vi "NewTS-ExecutionEngine.vi"() -> ()   [LabVIEW 2020]
uses:
  SubVIs/ExEng_TypeDefs.llb/ExcEng_TestCommand.ctl
  SubVIs/ExEng_TypeDefs.llb/ExecEng_LimitsType.ctl
  LabVIEW 2020 Toolkits/toolkits_lv2020_32bit/Synchronization.llb/SynchRefs_SetGet.ctl
  LabVIEW 2020 Toolkits/VI Server Toolkit/VI Server Libraries/VI Server_SetControl.llb/VI Server_1D_STR_Set.vi
  LabVIEW 2020 Toolkits/VI Server Toolkit/VI Server Libraries/VI Server_GetControl.llb/VI Server_1D_Array_STR_Get.vi
  LabVIEW 2020 Toolkits/VI Server Toolkit/VI Server Libraries/VI Server_SetControl.llb/VI Server_1D_U16_Set.vi
  LabVIEW 2020 Toolkits/VI Server Toolkit/VI Server Libraries/VI Server_GetControl.llb/VI Server_DBL_Get.vi
  LabVIEW 2020 Toolkits/VI Server Toolkit/VI Server Libraries/VI Server_Set Controls.llb/Set STR Control.vi
  LabVIEW 2020 Toolkits/VI Server Toolkit/VI Server Libraries/VI Server_GetControl.llb/VI Server_Bool_Get.vi
  LabVIEW 2020 Toolkits/VI Server Toolkit/VI Server Libraries/VI Server_SetControl.llb/VI Server_BOOL_Set.vi
  LabVIEW 2020 Toolkits/VI Server Toolkit/VI Server Libraries/VI Server_SetControl.llb/VI Server_DBL_Set.vi
  LabVIEW 2020 Toolkits/VI Server Toolkit/VI Server Libraries/VI Server_GetControl.llb/VI Server_STR_Get.vi
  LabVIEW 2020 Toolkits/VI Server Toolkit/VI Server Toolkit LV2013.lvlib
panel:
  in  "Test.PauseOnFailure":bool caption="Pause On Failure"
  in  "Test.Pause":bool
  in  "Test.Start":bool
  in  "EmergencyStop":bool
  in  "Test.ABORT":bool
  out "System.Message":string caption="System Message:"
  in  "Help":bool
  in  "EXIT":bool
  in  "Tab.Main":T1(tab)=enum."TEST EDITOR"
  out "Test.NumberOfJumps":i32 caption="Number Of Jumps"
  out "Test.Repeat.NumberOfFailures":i32 caption="Number Of Failures"
  out "Test.Repeat.RunOf":string caption="Test:Run"
  in  "SerialNumbers.Array":string[](array[string])=["sssss"] caption="Serial Numbers"
  out "Test.ElapsedTime":string="mm:ss" caption="Elapsed: Time"
  out "Test.Progress":u16(slide) caption="Progress" scale=0.0..100.0
  out "Messages & Status":string="Test Not Started"
  in  "Test.P/N":u16(ring)=4 caption="Part #" items=["BK Precision1696 Demo", "ExecEng Verification", "Execution Engive 2", "NewTS Video Demo", "NewTS Video Demo_1", "NI-USB6001", "NI-USB6343 Demo", "NI-USB6343 Demo MultiSlot", "NI-USB6525 Demo", "Operator Interface Demo", "PCIe-1760", "PIXCI-SV7", "SeaCOM-7203", "Slow drive", "SRS5330A Test", "USB 6343_test2", "USB6001 Test", "VECTOR 1610 Demo"]
  in  "Test.Tree":string[](tree) caption="Test"
  in  "TestCaseConfiguration_VisibleRow_Decr":bool
  in  "TestCaseConfiguration_VisibleRow_Incr":bool
  in  "CurrentInstruction":i32[](listbox)=[-1] caption="Current Instruction"
  in  "Test.EndTime":string caption="Test End Time"
  in  "Test.StartTime":string caption="Test Start Time"
  in  "Fixture.SlotSelector":u16(ring) caption="Fixture Slot Selector" items=["Slot 1"]
  out "TestCase.SAVE.Success":bool
  in  "TestCase.Update.Instruction":bool
  in  "TestCase.Add.Instruction":bool
  in  "TestCase.Execute.Instruction":bool
  in  "TestCase.SAVE":bool
  in  "TestCaseConfiguration":i32[](listbox)=[0] caption="Test Case Configuration"
  in  "Limits.Remove":bool
  in  "Limits.SAVE":bool
  in  "Limit.Units":string caption="Units"
  in  "Limit.Lo":dbl caption="Lo" format="%0.3f V"
  in  "Limit.Hi":dbl caption="Hi" format="%0.3f V"
  in  "LimitsIndex":u16=1 caption="Limits Index" min=1
  in  "TestCase.TraceLimits":bool
  in  "TestCase.StepDescription":string caption="Step Description:"
  out "TestCase.ExecutionTime":dbl caption="Execution Time:" format="%0.3f sec"
  in  "TestCase.Execute.Step.Pause":bool
  in  "TestCase.Execute.Steps":u16(ring) caption="Test Case: Pause After Step" items=["1.1", "1.2", "1.3", "1.4", "1.5", "1.6", "1.7", "1.8", "1.9", "1.10", "1.11", "1.12", "1.13", "1.14", "1.15", "1.16", "1.17", "1.18", "1.19", "1.20", "1.21", "1.22", "1.23", "1.24", "1.25", "1.26", "1.27", "1.28", "1.29", "1.30", "1.31"]
  in  "TestCase.Add.Instruction.Pos":bool
  in  "TestConfiguration.Run.Step":bool
  in  "TestCaseExecution.PauseOnFailure":bool caption="TestCaseExecution.StopOnFailure"
  out "TestConfiguration.Execute.Pass/Fail":bool caption="Tests: Pass/Fail"
  in  "Settings.P/N":u16(ring)=4 caption="Part #" items=["BK Precision1696 Demo", "ExecEng Verification", "Execution Engive 2", "NewTS Video Demo", "NewTS Video Demo_1", "NI-USB6001", "NI-USB6343 Demo", "NI-USB6343 Demo MultiSlot", "NI-USB6525 Demo", "Operator Interface Demo", "PCIe-1760", "PIXCI-SV7", "SeaCOM-7203", "Slow drive", "SRS5330A Test", "USB 6343_test2", "USB6001 Test", "VECTOR 1610 Demo"]
  in  "TestCase":u16(ring) caption="Test Case" items=["1", "1.1", "1.2", "1.3", "1.4", "2", "3"]
  in  "TestConfiguration.RunAll":bool
  in  "TestCase.Execute.Next":bool
  in  "TestCase.Execute.Pause":bool
  in  "TestCase.Execute.ABORT":bool
  in  "Performance.Verification.SAVE":bool
  in  "Performance.Verification.Pass/Fail":bool
  out "TestCase.Execute.Pass/Fail":bool caption="Test Case Instr. Execution"
  in  "TestCase.Execute.All":bool
  in  "TestCase.Execute.Selected":bool
  in  "TestCase.Execution.StepTime":u32 caption="Seq. Execution: Step Time" format="%d msec"
  in  "TestCase.InstrumentData.InRange":bool caption="In Range"
  in  "TestCase.Instrument.Data":dbl caption="MEASUREMENTS Num-DATA" format="%0.3f"
  in  "TestCase.LimitsIndex":u16(ring) caption="LIMITS INDEX" items=["101", "102"]
  in  "TestCase.Function.Argument3.DBL":dbl caption="ARGUMENT 3" format="%0.0f sec"
  in  "TestCase.Function.Argument3":u16(ring) caption="ARGUMENT 3"
  in  "TestCase.Function.Argument2":u16(ring) caption="ARGUMENT 2" items=["", "AI.Averaged.Mesurement", "Graph1", "Graph2", "DI.Line.State", "DO.Line.State.Verify", "DO.Port.State.Verify", "DI.Port.Lines.0:7", "DI.Port.Lines.8:15", "DI.Port.Lines.16:23", "DI.Port.Lines.24:31", "ctr0.In.Count", "ctr1.In.Count", "ctr2.In.Count", "ctr3.In.Count", "ctr0.Out.Frequency.Actual", "ctr0.Out.Duty Cycle.Actual", "ctr1.Out.Frequency.Actual", "ctr1.Out.Duty Cycle.Actual", "ctr2.Out.Frequency.Actual", "ctr2.Out.Duty Cycle.Actual", "ctr3.Out.Frequency.Actual", "ctr3.Out.Duty Cycle.Actual"]
  in  "TestCase.Function.Argument1":u16(ring) caption="ARGUMENT 1" items=["", "SET", "GET", "READ", "Wait For"]
  in  "TestCase.Function":u16(ring)=57 caption="INSTR/FUNCTION" items=["", "BK Precision 1696", "DPO2012B", "Data Processor", "E4443A Spectrum Analyzer", "EC-8200", "EXI-8000PCIe", "Keithley2100", "NAI5330A", "NAI8810A", "NI-USB6001", "NI-USB6212", "NI-USB6343", "NI-USB6509", "NI-USB6525", "PCIe-1760", "PEXHDCAP60L2", "PIXCI-SV7", "SWT", "SeaCOM-7203", "UDP Monitor", "VECTOR 1610", "-", "Execute Test Case Ones", "-", "ABORT on Failure", "Operator Message on Fail", "Operator Message on Pass", "-", "Jump", "Jump on Pass", "Jump on Fail", "-", "Local Jump", "Local Jump On Fail", "Local Jump On Pass", "-", "Jump: Number of Repeats", "Reset Jump Counter", "-", "Simple Message", "Operator's Input", "Operator's Input Pass/Fail", "Operator's Input/Test Failure", "Operator's Input/Pre-Test", "Operator's Input+Pic", "Operator's Instructions+Pic", "-", "<Wait For> Timeout", "Delay", "Delay Between Instructions", "Timer", "-", "Clear", "Export Graph to File", "-", "SAVE Num-Data to Memory", "SAVE Str-Data to Memory", "Copy NUM.Data to Arg.3", "-", "Load Num-Mem  from previos test", "Save Num-Mem at the test completion", "-", "RST Num-Data Memory", "RST Str-Data Memory", "-", "Save Start Time to Memory", "Save End Time to Memory", "-", "TEST END"]
  in  "TestCase.Parameter":string="AI0 & AO0 demo test" caption="PARAMETER"
  in  "TestCase.Conditions":string caption="TEST CONDITIONS"
  in  "TestCase.Description":string="AI0 & AO0 demo test" caption="DESCRIPTION"
  in  "TestConfiguration":i32[](listbox)=[0] caption="Test Configuration"
  in  "Limit.Message":string caption="Message"
  in  "TestCase.Function.Argument3.STR":string caption="ARGUMENT 3"
  in  "Limit.PicturePath":path caption="Picture Path"
  in  "TestCase.Instrument.Data.Str":string caption="MEASUREMENTS Str-DATA"
  in  "Graph2.Plots":u16(ring) items=["NI-USB6343/ai0", "NI-USB6343/ai1", "NI-USB6343/ai0"]
  in  "Graph1.Plots":u16(ring) items=["NI-USB6343/ai0", "NI-USB6343/ai1", "NI-USB6343/ai0"]
  out "Graph2":waveform(dbl)[](graph) caption="GRAPH 2"
  out "Graph1":waveform(dbl)[](graph) caption="GPAPH 1"
  out "Image3":picture caption="IMAGE 3"
  out "Image2":picture caption="IMAGE 2"
  out "Image1":picture caption="IMAGE 1"
  in  "NumMem.Tab":enum32{"MEM/Num1", "MEM/Num2"}(tab)
  in  "Mem176":dbl=nan format="%0.3f"
  in  "Mem175":dbl=nan format="%0.3f"
  in  "Mem174":dbl=nan format="%0.3f"
  in  "Mem173":dbl=nan format="%0.3f"
  in  "Mem172":dbl=nan format="%0.3f"
  in  "Mem171":dbl=nan format="%0.3f"
  in  "Mem170":dbl=nan format="%0.3f"
  in  "Mem169":dbl=nan format="%0.3f"
  in  "Mem168":dbl=nan format="%0.3f"
  in  "Mem167":dbl=nan format="%0.3f"
  in  "Mem166":dbl=nan format="%0.3f"
  in  "Mem165":dbl=nan format="%0.3f"
  in  "Mem164":dbl=nan format="%0.3f"
  in  "Mem163":dbl=nan format="%0.3f"
  in  "Mem162":dbl=nan format="%0.3f"
  in  "Mem161":dbl=nan format="%0.3f"
  in  "Mem80":dbl=nan format="%0.3f"
  in  "Mem79":dbl=nan format="%0.3f"
  in  "Mem78":dbl=nan format="%0.3f"
  in  "Mem77":dbl=nan format="%0.3f"
  in  "Mem76":dbl=nan format="%0.3f"
  in  "Mem75":dbl=nan format="%0.3f"
  in  "Mem74":dbl=nan format="%0.3f"
  in  "Mem73":dbl=nan format="%0.3f"
  in  "Mem72":dbl=nan format="%0.3f"
  in  "Mem71":dbl=nan format="%0.3f"
  in  "Mem70":dbl=nan format="%0.3f"
  in  "Mem69":dbl=nan format="%0.3f"
  in  "Mem68":dbl=nan format="%0.3f"
  in  "Mem67":dbl=nan format="%0.3f"
  in  "Mem66":dbl=nan format="%0.3f"
  in  "Mem65":dbl=nan format="%0.3f"
  in  "Mem160":dbl=nan format="%0.3f"
  in  "Mem159":dbl=nan format="%0.3f"
  in  "Mem158":dbl=nan format="%0.3f"
  in  "Mem157":dbl=nan format="%0.3f"
  in  "Mem156":dbl=nan format="%0.3f"
  in  "Mem155":dbl=nan format="%0.3f"
  in  "Mem154":dbl=nan format="%0.3f"
  in  "Mem153":dbl=nan format="%0.3f"
  in  "Mem152":dbl=nan format="%0.3f"
  in  "Mem151":dbl=nan format="%0.3f"
  in  "Mem150":dbl=nan format="%0.3f"
  in  "Mem149":dbl=nan format="%0.3f"
  in  "Mem148":dbl=nan format="%0.3f"
  in  "Mem147":dbl=nan format="%0.3f"
  in  "Mem146":dbl=nan format="%0.3f"
  in  "Mem145":dbl=nan format="%0.3f"
  in  "Mem64":dbl=nan format="%0.3f"
  in  "Mem63":dbl=nan format="%0.3f"
  in  "Mem62":dbl=nan format="%0.3f"
  in  "Mem61":dbl=nan format="%0.3f"
  in  "Mem60":dbl=nan format="%0.3f"
  in  "Mem59":dbl=nan format="%0.3f"
  in  "Mem58":dbl=nan format="%0.3f"
  in  "Mem57":dbl=nan format="%0.3f"
  in  "Mem56":dbl=nan format="%0.3f"
  in  "Mem55":dbl=nan format="%0.3f"
  in  "Mem54":dbl=nan format="%0.3f"
  in  "Mem53":dbl=nan format="%0.3f"
  in  "Mem52":dbl=nan format="%0.3f"
  in  "Mem51":dbl=nan format="%0.3f"
  in  "Mem50":dbl=nan format="%0.3f"
  in  "Mem49":dbl=nan format="%0.3f"
  in  "Mem144":dbl=nan format="%0.3f"
  in  "Mem143":dbl=nan format="%0.3f"
  in  "Mem142":dbl=nan format="%0.3f"
  in  "Mem141":dbl=nan format="%0.3f"
  in  "Mem140":dbl=nan format="%0.3f"
  in  "Mem139":dbl=nan format="%0.3f"
  in  "Mem138":dbl=nan format="%0.3f"
  in  "Mem137":dbl=nan format="%0.3f"
  in  "Mem136":dbl=nan format="%0.3f"
  in  "Mem135":dbl=nan format="%0.3f"
  in  "Mem134":dbl=nan format="%0.3f"
  in  "Mem133":dbl=nan format="%0.3f"
  in  "Mem132":dbl=nan format="%0.3f"
  in  "Mem131":dbl=nan format="%0.3f"
  in  "Mem130":dbl=nan format="%0.3f"
  in  "Mem129":dbl=nan format="%0.3f"
  in  "Mem48":dbl=nan format="%0.3f"
  in  "Mem47":dbl=nan format="%0.3f"
  in  "Mem46":dbl=nan format="%0.3f"
  in  "Mem45":dbl=nan format="%0.3f"
  in  "Mem44":dbl=nan format="%0.3f"
  in  "Mem43":dbl=nan format="%0.3f"
  in  "Mem42":dbl=nan format="%0.3f"
  in  "Mem41":dbl=nan format="%0.3f"
  in  "Mem40":dbl=nan format="%0.3f"
  in  "Mem39":dbl=nan format="%0.3f"
  in  "Mem38":dbl=nan format="%0.3f"
  in  "Mem37":dbl=nan format="%0.3f"
  in  "Mem36":dbl=nan format="%0.3f"
  in  "Mem35":dbl=nan format="%0.3f"
  in  "Mem34":dbl=nan format="%0.3f"
  in  "Mem33":dbl=nan format="%0.3f"
  in  "Mem128":dbl=nan format="%0.3f"
  in  "Mem127":dbl=nan format="%0.3f"
  in  "Mem126":dbl=nan format="%0.3f"
  in  "Mem125":dbl=nan format="%0.3f"
  in  "Mem124":dbl=nan format="%0.3f"
  in  "Mem123":dbl=nan format="%0.3f"
  in  "Mem122":dbl=nan format="%0.3f"
  in  "Mem121":dbl=nan format="%0.3f"
  in  "Mem120":dbl=nan format="%0.3f"
  in  "Mem119":dbl=nan format="%0.3f"
  in  "Mem118":dbl=nan format="%0.3f"
  in  "Mem117":dbl=nan format="%0.3f"
  in  "Mem116":dbl=nan format="%0.3f"
  in  "Mem115":dbl=nan format="%0.3f"
  in  "Mem114":dbl=nan format="%0.3f"
  in  "Mem113":dbl=nan format="%0.3f"
  in  "Mem32":dbl=nan format="%0.3f"
  in  "Mem31":dbl=nan format="%0.3f"
  in  "Mem30":dbl=nan format="%0.3f"
  in  "Mem29":dbl=nan format="%0.3f"
  in  "Mem28":dbl=nan format="%0.3f"
  in  "Mem27":dbl=nan format="%0.3f"
  in  "Mem26":dbl=nan format="%0.3f"
  in  "Mem25":dbl=nan format="%0.3f"
  in  "Mem24":dbl=nan format="%0.3f"
  in  "Mem23":dbl=nan format="%0.3f"
  in  "Mem22":dbl=nan format="%0.3f"
  in  "Mem21":dbl=nan format="%0.3f"
  in  "Mem20":dbl=nan format="%0.3f"
  in  "Mem19":dbl=nan format="%0.3f"
  in  "Mem18":dbl=nan format="%0.3f"
  in  "Mem17":dbl=nan format="%0.3f"
  in  "Mem112":dbl=nan format="%0.3f"
  in  "Mem111":dbl=nan format="%0.3f"
  in  "Mem110":dbl=nan format="%0.3f"
  in  "Mem109":dbl=nan format="%0.3f"
  in  "Mem108":dbl=nan format="%0.3f"
  in  "Mem107":dbl=nan format="%0.3f"
  in  "Mem106":dbl=nan format="%0.3f"
  in  "Mem105":dbl=nan format="%0.3f"
  in  "Mem104":dbl=nan format="%0.3f"
  in  "Mem103":dbl=nan format="%0.3f"
  in  "Mem102":dbl=nan format="%0.3f"
  in  "Mem101":dbl=nan format="%0.3f"
  in  "Mem100":dbl=nan format="%0.3f"
  in  "Mem99":dbl=nan format="%0.3f"
  in  "Mem98":dbl=nan format="%0.3f"
  in  "Mem97":dbl=nan format="%0.3f"
  in  "Mem16":dbl=nan format="%0.3f"
  in  "Mem15":dbl=nan format="%0.3f"
  in  "Mem14":dbl=120.0 format="%0.3f"
  in  "Mem13":dbl=90.0 format="%0.3f"
  in  "Mem12":dbl=44.999 format="%0.3f"
  in  "Mem11":dbl=48059.0 format="%0.3f"
  in  "Mem10":dbl=43690.0 format="%0.3f"
  in  "Mem9":dbl=nan format="%0.3f"
  in  "Mem8":dbl=nan format="%0.3f"
  in  "Mem7":dbl=nan format="%0.3f"
  in  "Mem6":dbl=nan format="%0.3f"
  in  "Mem5":dbl format="%0.3f"
  in  "Mem4":dbl=nan format="%0.3f"
  in  "Mem3":dbl=6.501 format="%0.3f P"
  in  "Mem2":dbl=149.833 format="%0.3f F"
  in  "Mem1":dbl=1.0 format="%0.3f P"
  in  "Mem192":dbl=nan format="%0.3f"
  in  "Mem191":dbl=nan format="%0.3f"
  in  "Mem190":dbl=nan format="%0.3f"
  in  "Mem189":dbl=nan format="%0.3f"
  in  "Mem188":dbl=nan format="%0.3f"
  in  "Mem187":dbl=nan format="%0.3f"
  in  "Mem186":dbl=nan format="%0.3f"
  in  "Mem185":dbl=nan format="%0.3f"
  in  "Mem184":dbl=nan format="%0.3f"
  in  "Mem183":dbl=nan format="%0.3f"
  in  "Mem182":dbl=nan format="%0.3f"
  in  "Mem181":dbl=nan format="%0.3f"
  in  "Mem180":dbl=nan format="%0.3f"
  in  "Mem179":dbl=nan format="%0.3f"
  in  "Mem178":dbl=nan format="%0.3f"
  in  "Mem177":dbl=nan format="%0.3f"
  in  "Mem96":dbl=nan format="%0.3f"
  in  "Mem95":dbl=nan format="%0.3f"
  in  "Mem94":dbl=nan format="%0.3f"
  in  "Mem93":dbl=nan format="%0.3f"
  in  "Mem92":dbl=nan format="%0.3f"
  in  "Mem91":dbl=nan format="%0.3f"
  in  "Mem90":dbl=nan format="%0.3f"
  in  "Mem89":dbl=nan format="%0.3f"
  in  "Mem88":dbl=nan format="%0.3f"
  in  "Mem87":dbl=nan format="%0.3f"
  in  "Mem86":dbl=nan format="%0.3f"
  in  "Mem85":dbl=nan format="%0.3f"
  in  "Mem84":dbl=nan format="%0.3f"
  in  "Mem83":dbl=nan format="%0.3f"
  in  "Mem82":dbl=nan format="%0.3f"
  in  "Mem81":dbl=nan format="%0.3f"
  in  "Mem203":dbl=nan format="%0.3f"
  in  "Mem208":dbl=nan format="%0.3f"
  in  "Mem207":dbl=120.0 format="%0.3f"
  in  "Mem206":dbl=90.0 format="%0.3f"
  in  "Mem205":dbl=44.999 format="%0.3f"
  in  "Mem204":dbl=48059.0 format="%0.3f"
  in  "Mem202":dbl=43690.0 format="%0.3f"
  in  "Mem201":dbl=nan format="%0.3f"
  in  "Mem200":dbl=nan format="%0.3f"
  in  "Mem199":dbl=nan format="%0.3f"
  in  "Mem198":dbl=nan format="%0.3f"
  in  "Mem197":dbl format="%0.3f"
  in  "Mem196":dbl=nan format="%0.3f"
  in  "Mem195":dbl=6.501 format="%0.3f"
  in  "Mem194":dbl=149.833 format="%0.3f"
  in  "Mem193":dbl=1.0 format="%0.3f"
  in  "Mem288":dbl=nan format="%0.3f"
  in  "Mem287":dbl=nan format="%0.3f"
  in  "Mem286":dbl=nan format="%0.3f"
  in  "Mem285":dbl=nan format="%0.3f"
  in  "Mem284":dbl=nan format="%0.3f"
  in  "Mem283":dbl=nan format="%0.3f"
  in  "Mem282":dbl=nan format="%0.3f"
  in  "Mem281":dbl=nan format="%0.3f"
  in  "Mem280":dbl=nan format="%0.3f"
  in  "Mem279":dbl=nan format="%0.3f"
  in  "Mem278":dbl=nan format="%0.3f"
  in  "Mem277":dbl=nan format="%0.3f"
  in  "Mem276":dbl=nan format="%0.3f"
  in  "Mem275":dbl=nan format="%0.3f"
  in  "Mem274":dbl=nan format="%0.3f"
  in  "Mem273":dbl=nan format="%0.3f"
  in  "Mem303":dbl=nan format="%0.3f"
  in  "Mem302":dbl=nan format="%0.3f"
  in  "Mem301":dbl=nan format="%0.3f"
  in  "Mem300":dbl=nan format="%0.3f"
  in  "Mem299":dbl=nan format="%0.3f"
  in  "Mem298":dbl=nan format="%0.3f"
  in  "Mem297":dbl=nan format="%0.3f"
  in  "Mem296":dbl=nan format="%0.3f"
  in  "Mem295":dbl=nan format="%0.3f"
  in  "Mem294":dbl=nan format="%0.3f"
  in  "Mem293":dbl=nan format="%0.3f"
  in  "Mem292":dbl=nan format="%0.3f"
  in  "Mem291":dbl=nan format="%0.3f"
  in  "Mem290":dbl=nan format="%0.3f"
  in  "Mem289":dbl=nan format="%0.3f"
  in  "Mem304":dbl=nan format="%0.3f"
  in  "Mem383":dbl=nan format="%0.3f"
  in  "Mem382":dbl=nan format="%0.3f"
  in  "Mem381":dbl=nan format="%0.3f"
  in  "Mem380":dbl=nan format="%0.3f"
  in  "Mem379":dbl=nan format="%0.3f"
  in  "Mem378":dbl=nan format="%0.3f"
  in  "Mem377":dbl=nan format="%0.3f"
  in  "Mem376":dbl=nan format="%0.3f"
  in  "Mem375":dbl=nan format="%0.3f"
  in  "Mem374":dbl=nan format="%0.3f"
  in  "Mem373":dbl=nan format="%0.3f"
  in  "Mem372":dbl=nan format="%0.3f"
  in  "Mem371":dbl=nan format="%0.3f"
  in  "Mem370":dbl=nan format="%0.3f"
  in  "Mem369":dbl=nan format="%0.3f"
  in  "Mem384":dbl=nan format="%0.3f"
  in  "Mem368":dbl=nan format="%0.3f"
  in  "Mem367":dbl=nan format="%0.3f"
  in  "Mem366":dbl=nan format="%0.3f"
  in  "Mem365":dbl=nan format="%0.3f"
  in  "Mem364":dbl=nan format="%0.3f"
  in  "Mem363":dbl=nan format="%0.3f"
  in  "Mem362":dbl=nan format="%0.3f"
  in  "Mem361":dbl=nan format="%0.3f"
  in  "Mem360":dbl=nan format="%0.3f"
  in  "Mem359":dbl=nan format="%0.3f"
  in  "Mem358":dbl=nan format="%0.3f"
  in  "Mem357":dbl=nan format="%0.3f"
  in  "Mem356":dbl=nan format="%0.3f"
  in  "Mem355":dbl=nan format="%0.3f"
  in  "Mem354":dbl=nan format="%0.3f"
  in  "Mem353":dbl=nan format="%0.3f"
  in  "Mem272":dbl=nan format="%0.3f"
  in  "Mem271":dbl=nan format="%0.3f"
  in  "Mem270":dbl=nan format="%0.3f"
  in  "Mem269":dbl=nan format="%0.3f"
  in  "Mem268":dbl=nan format="%0.3f"
  in  "Mem267":dbl=nan format="%0.3f"
  in  "Mem266":dbl=nan format="%0.3f"
  in  "Mem265":dbl=nan format="%0.3f"
  in  "Mem264":dbl=nan format="%0.3f"
  in  "Mem263":dbl=nan format="%0.3f"
  in  "Mem262":dbl=nan format="%0.3f"
  in  "Mem261":dbl=nan format="%0.3f"
  in  "Mem260":dbl=nan format="%0.3f"
  in  "Mem259":dbl=nan format="%0.3f"
  in  "Mem258":dbl=nan format="%0.3f"
  in  "Mem257":dbl=nan format="%0.3f"
  in  "Mem352":dbl=nan format="%0.3f"
  in  "Mem351":dbl=nan format="%0.3f"
  in  "Mem350":dbl=nan format="%0.3f"
  in  "Mem349":dbl=nan format="%0.3f"
  in  "Mem348":dbl=nan format="%0.3f"
  in  "Mem347":dbl=nan format="%0.3f"
  in  "Mem346":dbl=nan format="%0.3f"
  in  "Mem345":dbl=nan format="%0.3f"
  in  "Mem344":dbl=nan format="%0.3f"
  in  "Mem343":dbl=nan format="%0.3f"
  in  "Mem342":dbl=nan format="%0.3f"
  in  "Mem341":dbl=nan format="%0.3f"
  in  "Mem340":dbl=nan format="%0.3f"
  in  "Mem339":dbl=nan format="%0.3f"
  in  "Mem338":dbl=nan format="%0.3f"
  in  "Mem337":dbl=nan format="%0.3f"
  in  "Mem256":dbl=nan format="%0.3f"
  in  "Mem255":dbl=nan format="%0.3f"
  in  "Mem254":dbl=nan format="%0.3f"
  in  "Mem253":dbl=nan format="%0.3f"
  in  "Mem252":dbl=nan format="%0.3f"
  in  "Mem251":dbl=nan format="%0.3f"
  in  "Mem250":dbl=nan format="%0.3f"
  in  "Mem249":dbl=nan format="%0.3f"
  in  "Mem248":dbl=nan format="%0.3f"
  in  "Mem247":dbl=nan format="%0.3f"
  in  "Mem246":dbl=nan format="%0.3f"
  in  "Mem245":dbl=nan format="%0.3f"
  in  "Mem244":dbl=nan format="%0.3f"
  in  "Mem243":dbl=nan format="%0.3f"
  in  "Mem242":dbl=nan format="%0.3f"
  in  "Mem241":dbl=nan format="%0.3f"
  in  "Mem336":dbl=nan format="%0.3f"
  in  "Mem335":dbl=nan format="%0.3f"
  in  "Mem334":dbl=nan format="%0.3f"
  in  "Mem333":dbl=nan format="%0.3f"
  in  "Mem332":dbl=nan format="%0.3f"
  in  "Mem331":dbl=nan format="%0.3f"
  in  "Mem330":dbl=nan format="%0.3f"
  in  "Mem329":dbl=nan format="%0.3f"
  in  "Mem328":dbl=nan format="%0.3f"
  in  "Mem327":dbl=nan format="%0.3f"
  in  "Mem326":dbl=nan format="%0.3f"
  in  "Mem325":dbl=nan format="%0.3f"
  in  "Mem324":dbl=nan format="%0.3f"
  in  "Mem323":dbl=nan format="%0.3f"
  in  "Mem322":dbl=nan format="%0.3f"
  in  "Mem321":dbl=nan format="%0.3f"
  in  "Mem240":dbl=nan format="%0.3f"
  in  "Mem239":dbl=nan format="%0.3f"
  in  "Mem238":dbl=nan format="%0.3f"
  in  "Mem237":dbl=nan format="%0.3f"
  in  "Mem236":dbl=nan format="%0.3f"
  in  "Mem235":dbl=nan format="%0.3f"
  in  "Mem234":dbl=nan format="%0.3f"
  in  "Mem233":dbl=nan format="%0.3f"
  in  "Mem232":dbl=nan format="%0.3f"
  in  "Mem231":dbl=nan format="%0.3f"
  in  "Mem230":dbl=nan format="%0.3f"
  in  "Mem229":dbl=nan format="%0.3f"
  in  "Mem228":dbl=nan format="%0.3f"
  in  "Mem227":dbl=nan format="%0.3f"
  in  "Mem226":dbl=nan format="%0.3f"
  in  "Mem225":dbl=nan format="%0.3f"
  in  "Mem319":dbl=nan format="%0.3f"
  in  "Mem318":dbl=nan format="%0.3f"
  in  "Mem317":dbl=nan format="%0.3f"
  in  "Mem316":dbl=nan format="%0.3f"
  in  "Mem315":dbl=nan format="%0.3f"
  in  "Mem314":dbl=nan format="%0.3f"
  in  "Mem313":dbl=nan format="%0.3f"
  in  "Mem312":dbl=nan format="%0.3f"
  in  "Mem311":dbl=nan format="%0.3f"
  in  "Mem310":dbl=nan format="%0.3f"
  in  "Mem309":dbl=nan format="%0.3f"
  in  "Mem308":dbl=nan format="%0.3f"
  in  "Mem307":dbl=nan format="%0.3f"
  in  "Mem306":dbl=nan format="%0.3f"
  in  "Mem305":dbl=nan format="%0.3f"
  in  "Mem320":dbl=nan format="%0.3f"
  in  "Mem223":dbl=nan format="%0.3f"
  in  "Mem222":dbl=nan format="%0.3f"
  in  "Mem221":dbl=nan format="%0.3f"
  in  "Mem220":dbl=nan format="%0.3f"
  in  "Mem219":dbl=nan format="%0.3f"
  in  "Mem218":dbl=nan format="%0.3f"
  in  "Mem217":dbl=nan format="%0.3f"
  in  "Mem216":dbl=nan format="%0.3f"
  in  "Mem215":dbl=nan format="%0.3f"
  in  "Mem214":dbl=nan format="%0.3f"
  in  "Mem213":dbl=nan format="%0.3f"
  in  "Mem212":dbl=nan format="%0.3f"
  in  "Mem211":dbl=nan format="%0.3f"
  in  "Mem210":dbl=nan format="%0.3f"
  in  "Mem209":dbl=nan format="%0.3f"
  in  "Mem224":dbl=nan format="%0.3f"
  in  "NumMem.FailedUpdates":i32(listbox) caption="NumMem: Failed Updates"
  in  "MEM.SAVE.AtTestCompletion":bool caption="MEM.RST.AtTestStart"
  in  "Num.Memory.LOAD":bool
  in  "Num.Memory.SAVE":bool
  in  "Num.Memory.FilePath":path caption="Num. Memory: FilePath"
  in  "MEM.RST.AtTestStart":bool
  in  "Mem.RST":bool
  in  "Test.End.DateTime":string caption="Test End: Date/Time"
  in  "Test.Start.DateTime":string caption="Test Start: Date/Time"
  in  "Mem.Str192":string caption="Mem192"
  in  "Mem.Str191":string caption="Mem191"
  in  "Mem.Str190":string caption="Mem190"
  in  "Mem.Str189":string caption="Mem189"
  in  "Mem.Str188":string caption="Mem188"
  in  "Mem.Str187":string caption="Mem187"
  in  "Mem.Str186":string caption="Mem186"
  in  "Mem.Str185":string caption="Mem185"
  in  "Mem.Str184":string caption="Mem184"
  in  "Mem.Str183":string caption="Mem183"
  in  "Mem.Str182":string caption="Mem182"
  in  "Mem.Str181":string caption="Mem181"
  in  "Mem.Str180":string caption="Mem180"
  in  "Mem.Str179":string caption="Mem179"
  in  "Mem.Str178":string caption="Mem178"
  in  "Mem.Str177":string caption="Mem177"
  in  "Mem.Str175":string caption="Mem176"
  in  "Mem.Str175 2":string caption="Mem175"
  in  "Mem.Str174":string caption="Mem174"
  in  "Mem.Str173":string caption="Mem173"
  in  "Mem.Str172":string caption="Mem172"
  in  "Mem.Str171":string caption="Mem171"
  in  "Mem.Str170":string caption="Mem170"
  in  "Mem.Str169":string caption="Mem169"
  in  "Mem.Str168":string caption="Mem168"
  in  "Mem.Str167":string caption="Mem167"
  in  "Mem.Str166":string caption="Mem166"
  in  "Mem.Str165":string caption="Mem165"
  in  "Mem.Str164":string caption="Mem164"
  in  "Mem.Str163":string caption="Mem163"
  in  "Mem.Str162":string caption="Mem162"
  in  "Mem.Str161":string caption="Mem161"
  in  "Mem.Str160":string caption="Mem160"
  in  "Mem.Str159":string caption="Mem159"
  in  "Mem.Str158":string caption="Mem158"
  in  "Mem.Str157":string caption="Mem157"
  in  "Mem.Str156":string caption="Mem156"
  in  "Mem.Str155":string caption="Mem155"
  in  "Mem.Str154":string caption="Mem154"
  in  "Mem.Str153":string caption="Mem153"
  in  "Mem.Str152":string caption="Mem152"
  in  "Mem.Str151":string caption="Mem151"
  in  "Mem.Str150":string caption="Mem150"
  in  "Mem.Str149":string caption="Mem149"
  in  "Mem.Str148":string caption="Mem148"
  in  "Mem.Str147":string caption="Mem147"
  in  "Mem.Str146":string caption="Mem146"
  in  "Mem.Str145":string caption="Mem145"
  in  "Mem.Str144":string caption="Mem144"
  in  "Mem.Str143":string caption="Mem143"
  in  "Mem.Str142":string caption="Mem142"
  in  "Mem.Str141":string caption="Mem141"
  in  "Mem.Str140":string caption="Mem140"
  in  "Mem.Str139":string caption="Mem139"
  in  "Mem.Str138":string caption="Mem138"
  in  "Mem.Str137":string caption="Mem137"
  in  "Mem.Str136":string caption="Mem136"
  in  "Mem.Str135":string caption="Mem135"
  in  "Mem.Str134":string caption="Mem134"
  in  "Mem.Str133":string caption="Mem133"
  in  "Mem.Str132":string caption="Mem132"
  in  "Mem.Str131":string caption="Mem131"
  in  "Mem.Str130":string caption="Mem130"
  in  "Mem.Str129":string caption="Mem129"
  in  "Mem.Str128":string caption="Mem128"
  in  "Mem.Str127":string caption="Mem127"
  in  "Mem.Str126":string caption="Mem126"
  in  "Mem.Str125":string caption="Mem125"
  in  "Mem.Str124":string caption="Mem124"
  in  "Mem.Str123":string caption="Mem123"
  in  "Mem.Str122":string caption="Mem122"
  in  "Mem.Str121":string caption="Mem121"
  in  "Mem.Str120":string caption="Mem120"
  in  "Mem.Str119":string caption="Mem119"
  in  "Mem.Str118":string caption="Mem118"
  in  "Mem.Str117":string caption="Mem117"
  in  "Mem.Str116":string caption="Mem116"
  in  "Mem.Str115":string caption="Mem115"
  in  "Mem.Str114":string caption="Mem114"
  in  "Mem.Str113":string caption="Mem113"
  in  "Mem.Str112":string caption="Mem112"
  in  "Mem.Str111":string caption="Mem111"
  in  "Mem.Str110":string caption="Mem110"
  in  "Mem.Str109":string caption="Mem109"
  in  "Mem.Str108":string caption="Mem108"
  in  "Mem.Str107":string caption="Mem107"
  in  "Mem.Str106":string caption="Mem106"
  in  "Mem.Str105":string caption="Mem105"
  in  "Mem.Str104":string caption="Mem104"
  in  "Mem.Str103":string caption="Mem103"
  in  "Mem.Str102":string caption="Mem102"
  in  "Mem.Str101":string caption="Mem101"
  in  "Mem.Str100":string caption="Mem100"
  in  "Mem.Str99":string caption="Mem99"
  in  "Mem.Str98":string caption="Mem98"
  in  "Mem.Str97":string caption="Mem97"
  in  "Mem.Str96":string caption="Mem96"
  in  "Mem.Str95":string caption="Mem95"
  in  "Mem.Str94":string caption="Mem94"
  in  "Mem.Str93":string caption="Mem93"
  in  "Mem.Str92":string caption="Mem92"
  in  "Mem.Str91":string caption="Mem91"
  in  "Mem.Str90":string caption="Mem90"
  in  "Mem.Str89":string caption="Mem89"
  in  "Mem.Str88":string caption="Mem88"
  in  "Mem.Str87":string caption="Mem87"
  in  "Mem.Str86":string caption="Mem86"
  in  "Mem.Str85":string caption="Mem85"
  in  "Mem.Str84":string caption="Mem84"
  in  "Mem.Str83":string caption="Mem83"
  in  "Mem.Str82":string caption="Mem82"
  in  "Mem.Str81":string caption="Mem81"
  in  "Mem.Str80":string caption="Mem80"
  in  "Mem.Str79":string caption="Mem79"
  in  "Mem.Str78":string caption="Mem78"
  in  "Mem.Str77":string caption="Mem77"
  in  "Mem.Str76":string caption="Mem76"
  in  "Mem.Str75":string caption="Mem75"
  in  "Mem.Str74":string caption="Mem74"
  in  "Mem.Str73":string caption="Mem73"
  in  "Mem.Str72":string caption="Mem72"
  in  "Mem.Str71":string caption="Mem71"
  in  "Mem.Str70":string caption="Mem70"
  in  "Mem.Str69":string caption="Mem69"
  in  "Mem.Str68":string caption="Mem68"
  in  "Mem.Str67":string caption="Mem67"
  in  "Mem.Str66":string caption="Mem66"
  in  "Mem.Str65":string caption="Mem65"
  in  "Mem.Str64":string caption="Mem64"
  in  "Mem.Str63":string caption="Mem63"
  in  "Mem.Str62":string caption="Mem62"
  in  "Mem.Str61":string caption="Mem61"
  in  "Mem.Str60":string caption="Mem60"
  in  "Mem.Str59":string caption="Mem59"
  in  "Mem.Str58":string caption="Mem58"
  in  "Mem.Str57":string caption="Mem57"
  in  "Mem.Str56":string caption="Mem56"
  in  "Mem.Str55":string caption="Mem55"
  in  "Mem.Str54":string caption="Mem54"
  in  "Mem.Str53":string caption="Mem53"
  in  "Mem.Str52":string caption="Mem52"
  in  "Mem.Str51":string caption="Mem51"
  in  "Mem.Str50":string caption="Mem50"
  in  "Mem.Str49":string caption="Mem49"
  in  "Mem.Str48":string caption="Mem48"
  in  "Mem.Str47":string caption="Mem47"
  in  "Mem.Str46":string caption="Mem46"
  in  "Mem.Str45":string caption="Mem45"
  in  "Mem.Str44":string caption="Mem44"
  in  "Mem.Str43":string caption="Mem43"
  in  "Mem.Str42":string caption="Mem42"
  in  "Mem.Str41":string caption="Mem41"
  in  "Mem.Str40":string caption="Mem40"
  in  "Mem.Str39":string caption="Mem39"
  in  "Mem.Str38":string caption="Mem38"
  in  "Mem.Str37":string caption="Mem37"
  in  "Mem.Str36":string caption="Mem36"
  in  "Mem.Str35":string caption="Mem35"
  in  "Mem.Str34":string caption="Mem34"
  in  "Mem.Str33":string caption="Mem33"
  in  "Mem.Str32":string caption="Mem32"
  in  "Mem.Str31":string caption="Mem31"
  in  "Mem.Str30":string caption="Mem30"
  in  "Mem.Str29":string caption="Mem29"
  in  "Mem.Str28":string caption="Mem28"
  in  "Mem.Str27":string caption="Mem27"
  in  "Mem.Str26":string caption="Mem26"
  in  "Mem.Str25":string caption="Mem25"
  in  "Mem.Str24":string caption="Mem24"
  in  "Mem.Str23":string caption="Mem23"
  in  "Mem.Str22":string caption="Mem22"
  in  "Mem.Str21":string caption="Mem21"
  in  "Mem.Str20":string caption="Mem20"
  in  "Mem.Str19":string caption="Mem19"
  in  "Mem.Str18":string caption="Mem18"
  in  "Mem.Str17":string caption="Mem17"
  in  "Mem.Str16":string caption="Mem16"
  in  "Mem.Str15":string caption="Mem15"
  in  "Mem.Str14":string caption="Mem14"
  in  "Mem.Str13":string caption="Mem13"
  in  "Mem.Str12":string caption="Mem12"
  in  "Mem.Str11":string caption="Mem11"
  in  "Mem.Str10":string caption="Mem10"
  in  "Mem.Str9":string caption="Mem9"
  in  "Mem.Str1 8":string caption="Mem8"
  in  "Mem.Str7":string caption="Mem7"
  in  "Mem.Str6":string caption="Mem6"
  in  "Mem.Str5":string caption="Mem5"
  in  "Mem.Str4":string caption="Mem4"
  in  "Mem.Str3":string caption="Mem3"
  in  "Mem.Str2":string caption="Mem2"
  in  "Mem.Str1":string caption="Mem1"
  in  "Mem.Str.RST":bool caption="Mem.RST"
  in  "Report.PDF.OpenWithACROBAT":bool
  in  "Report.PDF.File.Content.Clear":bool
  in  "Report.PDF.File.Read":bool
  in  "Report.PDF.Files":path[](array[path]) caption="Report PDF Files"
  out "Report.PDF.File.Content":string caption="Report Content"
  in  "Settings":enum32{"Communication", "Options"}(tab)
  in  "EmergencyStop.TEST":bool
  in  "EmergencyStop.LOAD":bool
  in  "EmergencyStop.SAVE":bool
  in  "EmergencyStop.Sequence":string[](array[string]) caption="EmergencyStop Sequence"
  in  "UDP.Responce.Array.EmptyAtStart":bool=TRUE caption="Performance.Verification.Enable"
  in  "TestCase.Diagnostics.Instruction":bool caption="TestCase.Execute.Instruction"
  in  "TestCase.Diagnostics.Next":bool
  in  "TestCase.Diagnostics.Pause":bool caption="TestCase.Execute.Pause"
  in  "TestCase.Diagnostics.ABORT":bool caption="TestCase.Execute.ABORT"
  out "UDP.Responce.Array":string[](array[string]) caption="UDP: Read"
  in  "UDP.Write.Array":string[](array[string]) caption="UDP: Write"
  in  "UDP.Test.String2.Send":bool caption="UDP.Test.String.Send"
  in  "UDP.Test.String2":string="DPO2012B::SET::FP.Hide::ON" caption="UDP: Test String"
  out "UDP.Sent.String":string="NAI8810A::SET::EXIT" caption="UDP: Sent String"
  in  "UDP.Responce.String.Monitor":bool=TRUE
  out "UDP.Responce.String":string="NAI8810A::SET::EXIT::ACK" caption="UDP: Responce String"
  in  "Instr.Responce.Timeout":u32=2000 caption="Instr. Responce Timeout" format="%d msec"
  in  "UDP.Test.String.Send":bool
  in  "UDP.Test.String":string="DPO2012B::GET::*IDN?" caption="UDP: Test String"
  in  "UDP.Port.RT":u16=58432 caption="UDP: Port.RT"
  in  "UDP.Port.BC":u16=58433 caption="UDP: Port.BC"
  in  "UDP.LocalPort":u16=58431 caption="UDP: Local Port"
  in  "UDP.IP.Address":string="234.5.6.7" caption="UDP: IP Address"
  out "Limits.List":u16[](array[numeric]) caption="Limits List"
  in  "Test.Results.LogFile.Folder":path caption="Test Results Log File Folder"
  in  "NotePad.Path":path=path "C:/Windows/notepad.exe" caption="Notepad Path"
  out "error out":errorcluster
  in  "Setup.AdobeAcrobat.Path":path caption="Adobe Acrobat Path"
  in  "TestExecution.PauseInInstrumentsFailure":bool
  in  "Test.Report.KeepMSWordReport":bool caption="Keep MS Word Report"
  in  "Test.Report.ContainsImages":bool caption="Contains Images"
  in  "Test.Report.DOCX-to-PDF.CMD":bool=TRUE caption="PDF Conversion"
  in  "Test.Report.ConvertToPDF":bool=TRUE caption="Performance.Verification.Enable"
  in  "Test.Report.Type":bool=TRUE caption="Report Template Type"
  in  "Test.Report.Skip":bool=TRUE caption="Performance.Verification.Enable"
  in  "Report.Test":bool
  in  "SimulateTestFailure":bool
  in  "NumMemory.Blinking":bool caption="NumMemory"
  in  "Limits.Table":i32[](listbox) caption="Limits Table"
  in  "Graph.SAVE.Format":bool caption="Graph SAVE Format"
  in  "Help.Enable":bool=TRUE caption="Performance.Verification.Enable"
  in  "TestTree.CollapseItems":bool=TRUE caption="Performance.Verification.Enable"
  in  "InstrumentLoad.Disable":bool=TRUE
  in  "Performance.Verification.Enable":bool
  in  "Test.Instruments.FP":bool=TRUE caption="Performance.Verification.Enable"
  in  "Jump.MAX.Number":i32=1000 caption="MAX Number of Jumps" min=1
  in  "Test.Repeat.NumberOf":i32=1000 caption="Number Of Repeats" min=1
  in  "Fixture.Slot8":bool caption="Slot 8"
  in  "Fixture.Slot7":bool caption="Slot 7"
  in  "Fixture.Slot6":bool caption="Slot 6"
  in  "Fixture.Slot5":bool caption="Slot 5"
  in  "Fixture.Slot4":bool caption="Slot 4"
  in  "Fixture.Slot3":bool caption="Slot 3"
  in  "Fixture.Slot2":bool caption="Slot 2"
  in  "Fixture.Slot1":bool caption="Slot 1"
  in  "TestExecution.DoNotCheckInstrument":bool
  in  "User.Password":string caption="Password"
  in  "Users.Level":u16(ring) caption="Level" items=["Operator", "Engineer", "Administrator"]
  in  "Users.Name":string caption="Name"
  in  "User.SAVE":bool
  in  "Users.Load":bool
  in  "User.Remove":bool
  in  "User.AddNew":bool
  in  "Users":i32(listbox)
  out "Instruments.Status":bool
  out "Login.Name":string="b" caption="Login Name"
  out "Login.Level":string="Engineer"
  in  "error in":errorcluster
  # "24NOV2023 build 2"
  # "M"
  # "M"
  # "M"
  # "M"
  # "M"
  # "M"
  # "M"
  # "LIMITS EDITOR"
  # "M"
  # "M"
  # "M"
  # "Verification"
  # "NOTE:\nThe format string (P or F) demotes Pass or Fail conditions.\n\nAll \"Memory\" controls have the user menu."
  # "NOTE:\nIf string contains (//P or //F)\nit demotes Pass or Fail conditions."
  # "M"
  # "UDP Tables"
  # "M"
  # "Multicast IP addresses must be in the 224.0.0.0 to 239.255.255.255 range."
  # "Verification Record"
  # "Istruments Loading"
  # "Test Tree"
  # "Online Help"
  # "Instruments FP"
  # "Report"
  # "M"
  # "Test Repeat"
  # "Test Fixture"
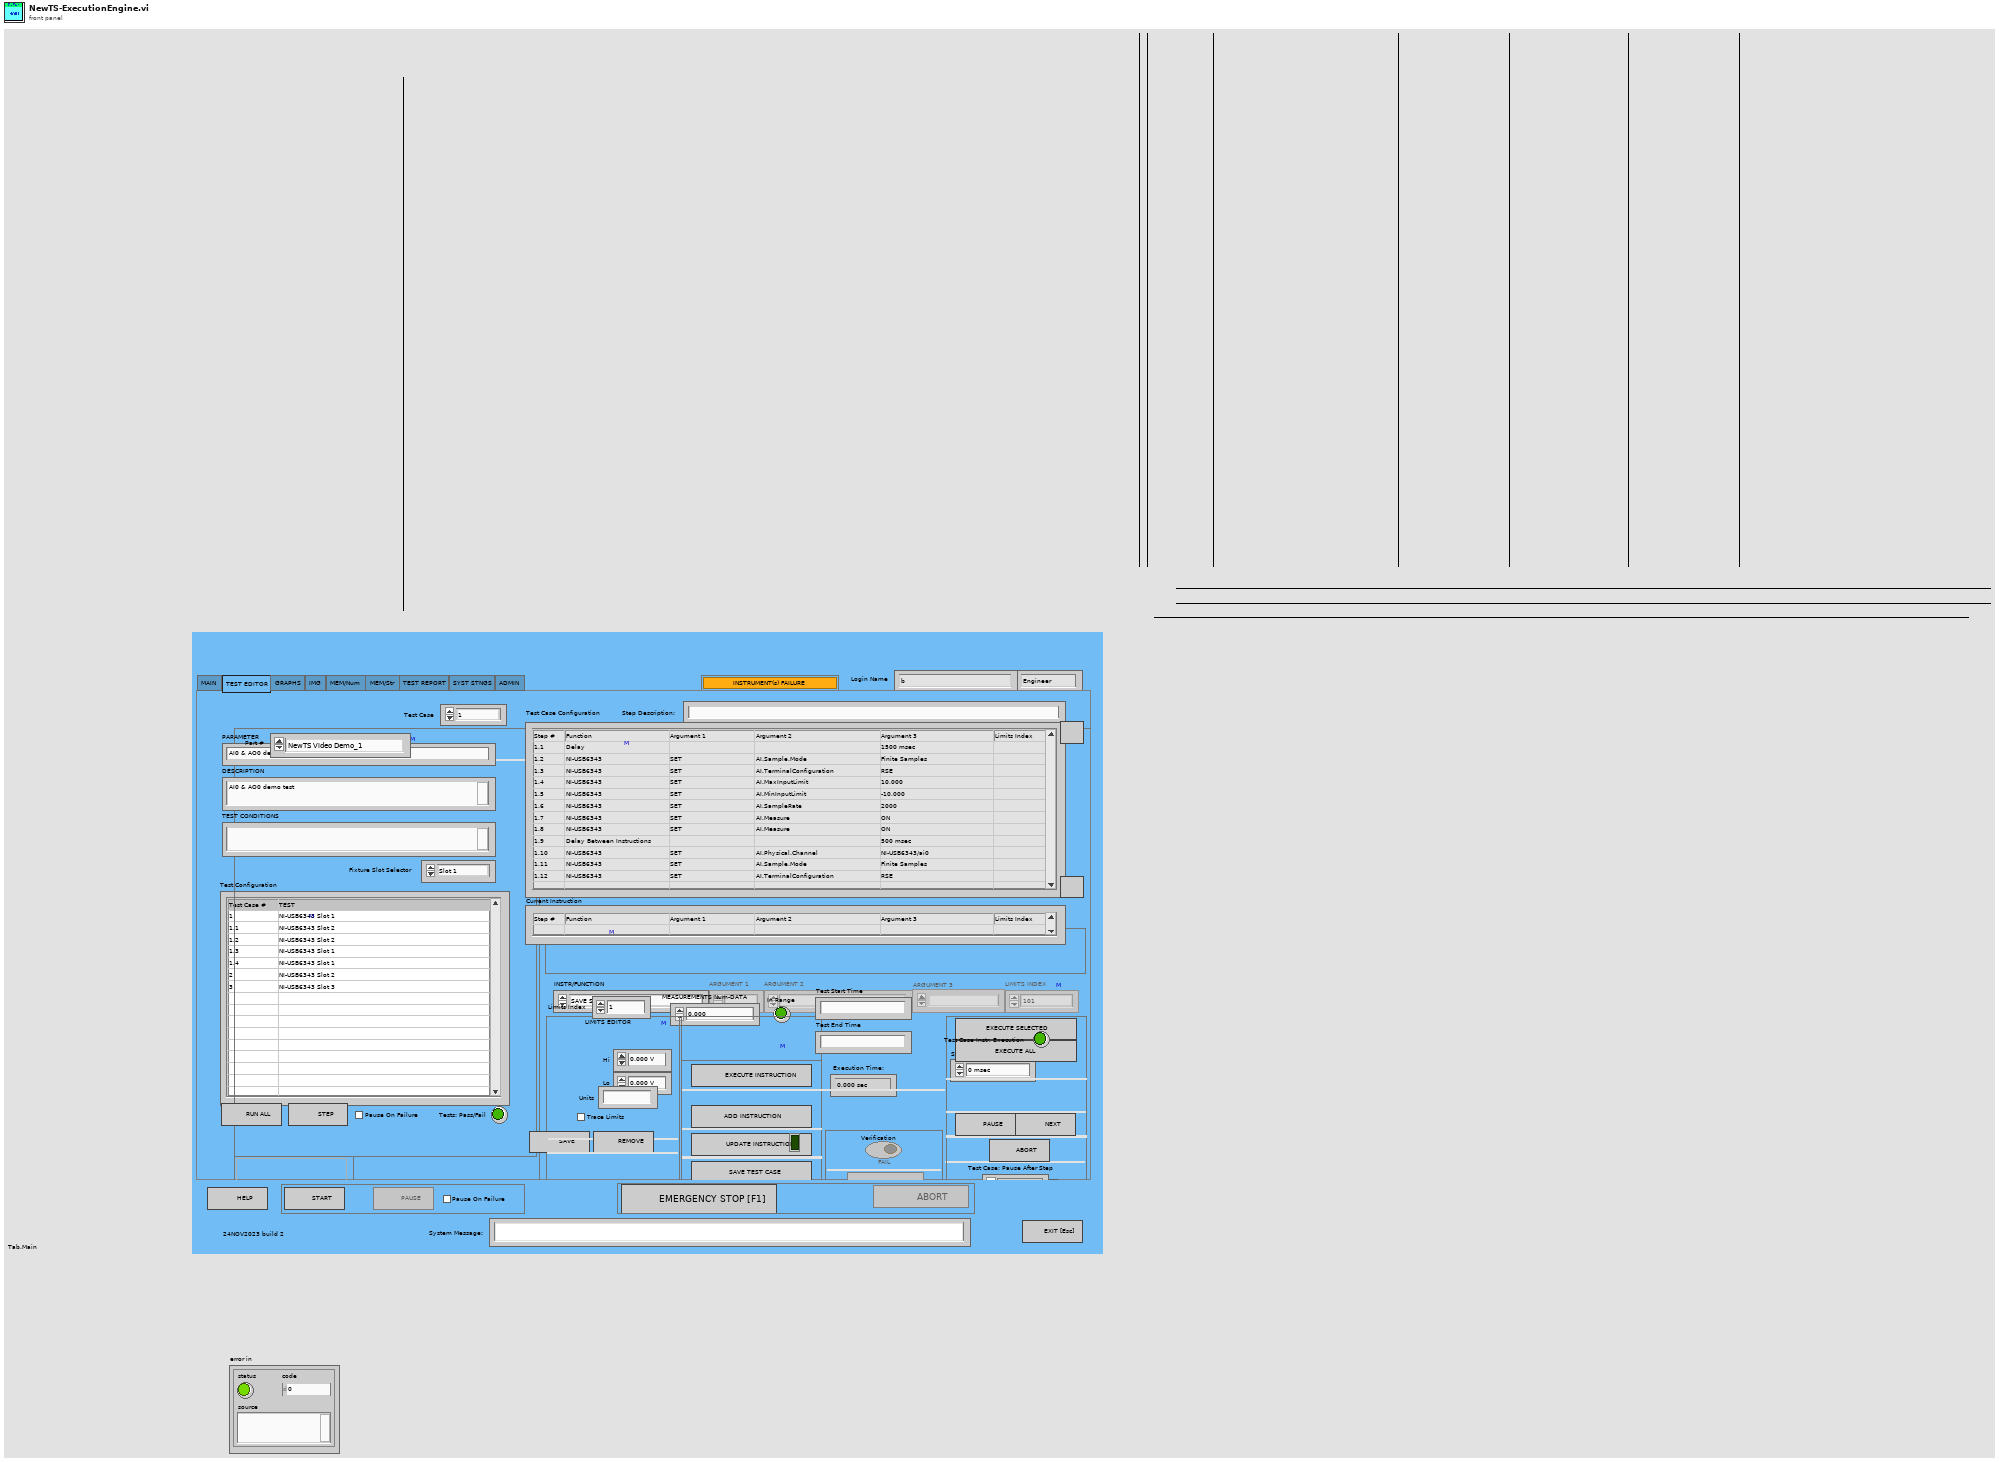
[diagram p1: front panel]
types:
  T1 = enum32{"MAIN", "TEST EDITOR", "GRAPHS", "IMG", "MEM/Num", "MEM/Str", "TEST REPORT", "SYST STNGS", "ADMIN"}
  T2 = enum8{"Enabled", "Disabled", "Disabled and Grayed Out"}
  T3 = typedef "VI Server_RefsCluster.ctl" = cluster{"Labels":string[], "Refs":refnum<vi>[], "VI Ref":refnum<vi>}
  T4 = typedef "ExcEng_TestCommand.ctl" = enum16{"", "Execute.Selected", "Execute.All", "Execute.Instruction", "TestConfiguration.RunAll", "TestConfiguration.Run.Step", "Test.Start", "Settings.P/N", "Execute Instruction"}
  T5 = typedef "ExecEng_LimitsType.ctl" = enum16{"STR", "DBL", "PATH"}
  T6 = typedef "SynchRefs_SetGet.ctl" = enum16{"Set", "Get"}
  T7 = cluster{"Color":u32, "PointStyle":u8, "LineStyle":u8, "Interp":u8, "LineWidth":u8, "BarPlotStyle":u8, "FillTo":i16, "XScaleIdx":u32, "YScaleIdx":u32, "Anti-Aliased":bool, "LabelFormat":u8, "TransitionType":u8, "TransitionLocation":u8, "DigitalLineStyle":u8}
  T8 = typedef "LVRowAndColumnUnsignedTypeDef.ctl" = cluster{"Row":u32, "Column":u32}
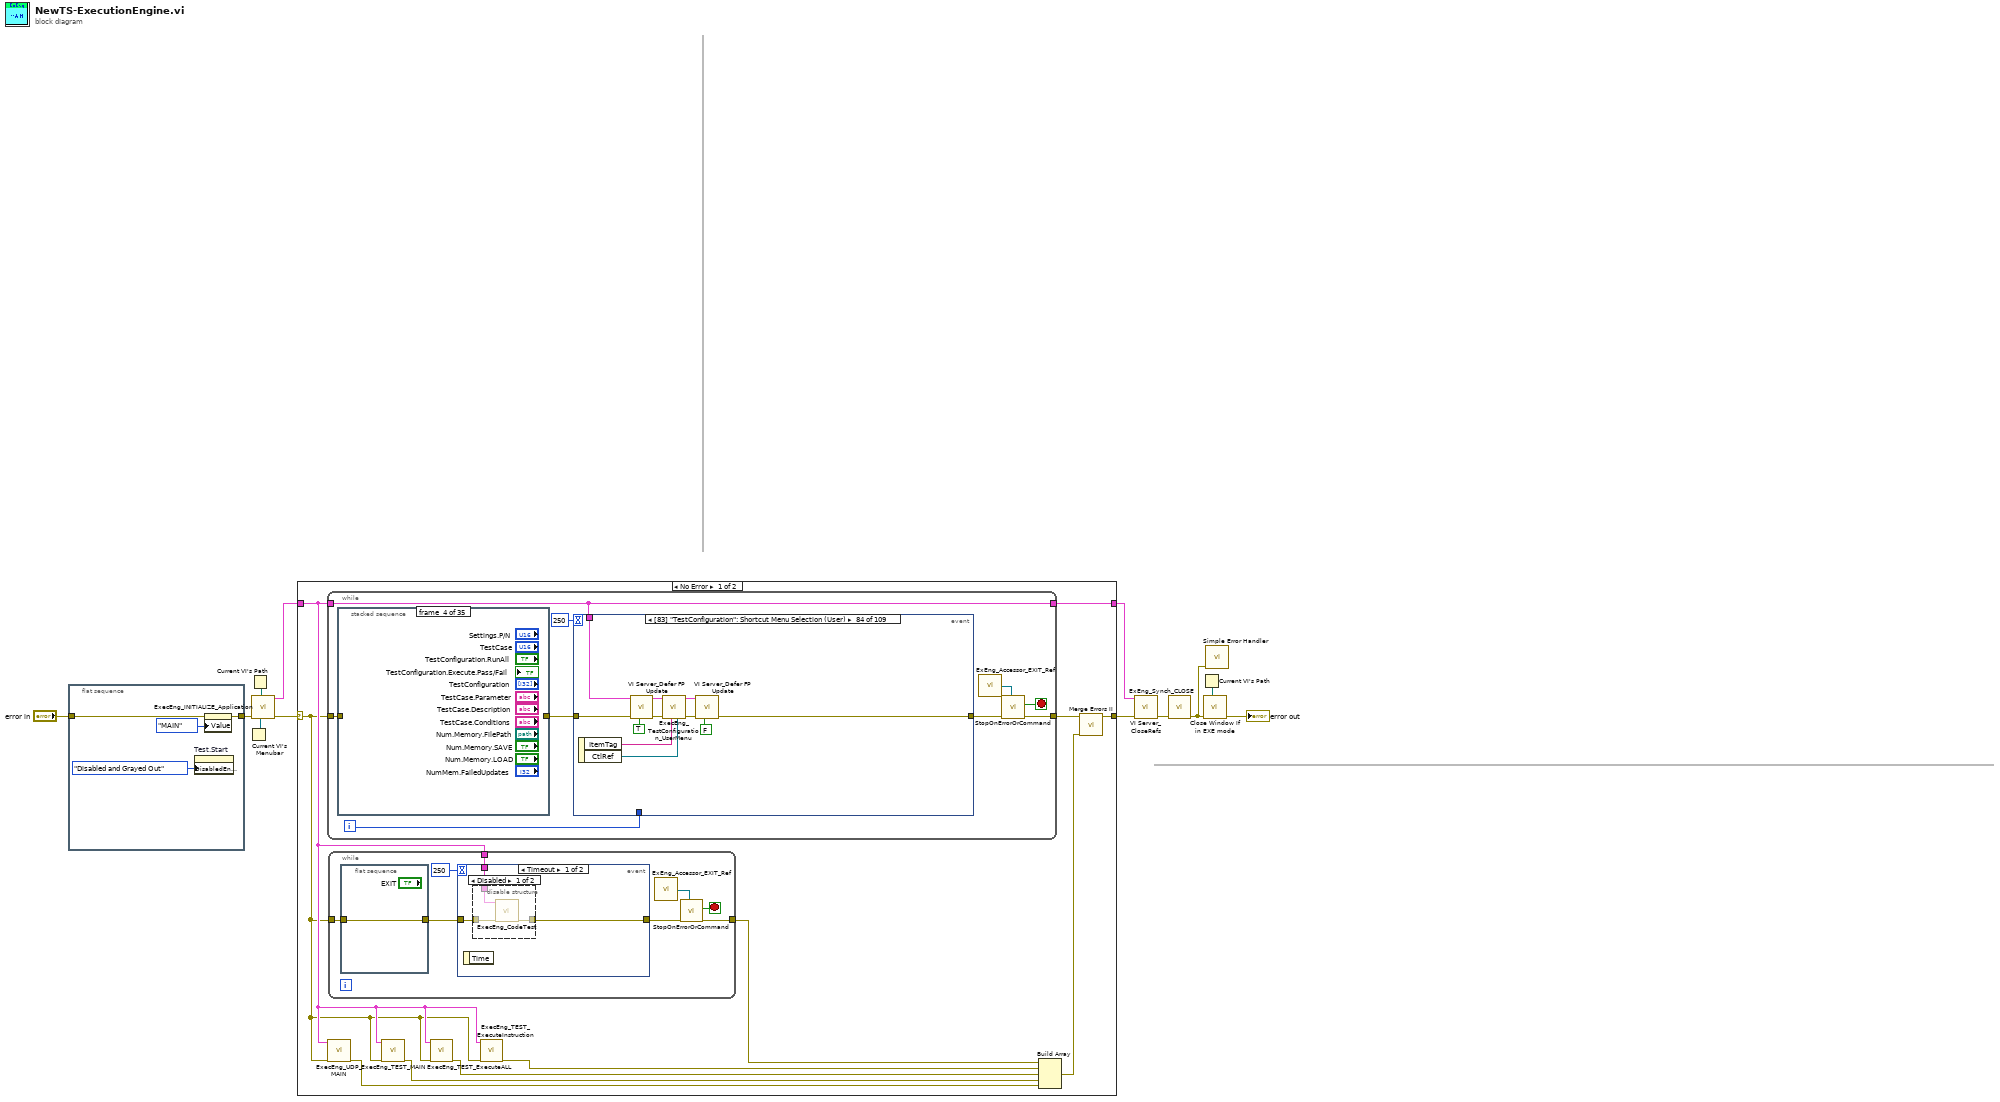
[diagram p0: block diagram]
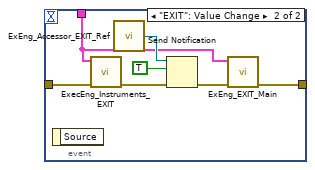
[diagram p3: hidden frame]
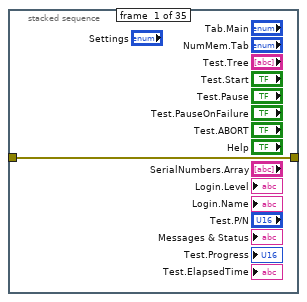
[diagram p4: hidden frame]
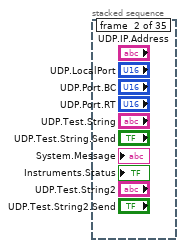
[diagram p5: hidden frame]
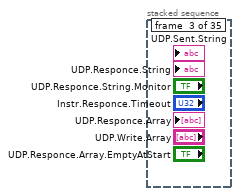
[diagram p6: hidden frame]
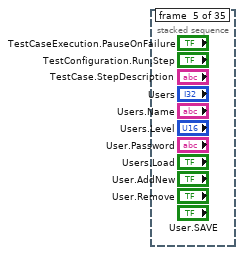
[diagram p7: hidden frame]
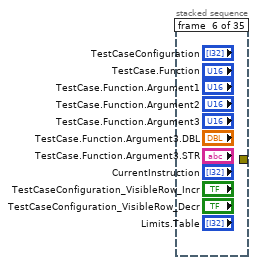
[diagram p8: hidden frame]
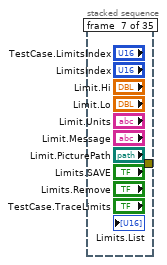
[diagram p9: hidden frame]
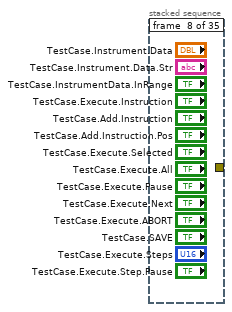
[diagram p10: hidden frame]
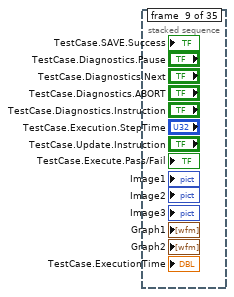
[diagram p11: hidden frame]
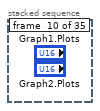
[diagram p12: hidden frame]
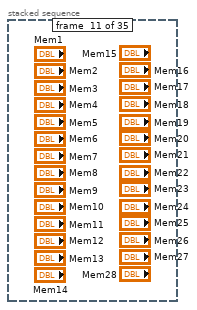
[diagram p13: hidden frame]
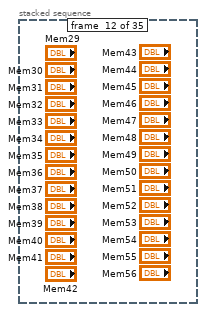
[diagram p14: hidden frame]
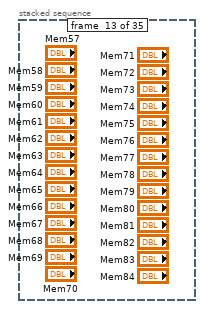
[diagram p15: hidden frame]
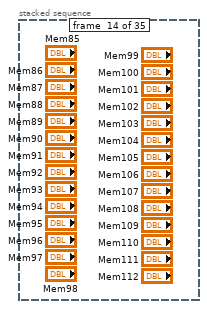
[diagram p16: hidden frame]
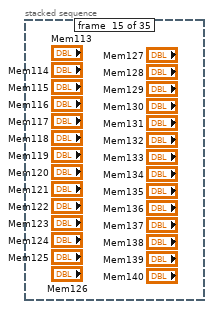
[diagram p17: hidden frame]
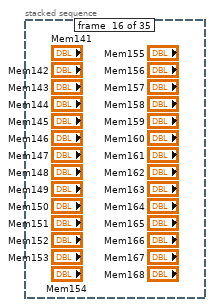
[diagram p18: hidden frame]
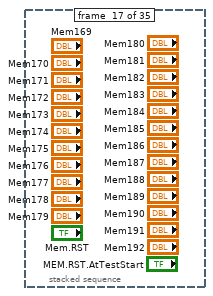
[diagram p19: hidden frame]
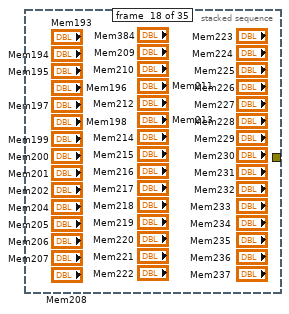
[diagram p20: hidden frame]
diagram:
  n1 = flat-sequence {
    tunnel: "error in" -> [w16]
    tunnel: [w15] -> w7
    frame #0 {
      n2 = property on="Test.Start" class="Bool (strict)"("DisabledEnum"=T2."Disabled and Grayed Out" ("Disabled")) -> ()  [unwired: 2 in, 2 out]
      n3 = property on="Tab.Main" class="TabCtl (strict)"(error in=w16, "Value"=T1."MAIN" ("Tab.Main")) -> (error out=w15:errorcluster)  [unwired: 1 in, 1 out]
    }
  }
  n4 = Current VI's Menubar() -> (w2:refnum<k9>)
  n5 = Current VI's Path() -> (path=w3:path)
  n6 = call "ExecEng_INITIALIZE_Application.vi"("menu reference"=w2, "TopVI Path"=w3, "error in (no error)"=w7) -> ("error out"=w11:errorcluster, "VI Server.RefsCluster.OUT"=w10:T3)  [unwired: 7 in]
  n7 = case shown="No Error" w11 {
    selector: w11 -> [w19 w785]
    tunnel: [w25 w785] -> w1
    tunnel: w10 -> [w20 _]
    tunnel: [w27 _] -> w9
    frame No Error {
      n8 = while {
        tunnel: w19 -> [w59]
        tunnel: [w57] -> w26
        tunnel: w20 -> [w53]
        tunnel: [w53] -> w27
        i -> [w52]
        stop <- w55 stop-if-true
        n9 = stacked-sequence {
          tunnel: w59 -> [w60 _ _ _ _ _ _ _ _ _ _ _ _ _ _ _ _ _ _ _ _ _ _ _ _ _ _ _ _ _ _ _ _ _ _]
          tunnel: [w60 _ _ _ _ _ _ _ _ _ _ _ _ _ _ _ _ _ _ _ _ _ _ _ _ _ _ _ _ _ _ _ _ _ _] -> w58
          frame #0 {
          }
          frame #1 {
          }
          frame #2 {
          }
          frame #3 {
          }
          frame #4 {
          }
          frame #5 {
          }
          frame #6 {
          }
          frame #7 {
          }
          frame #8 {
          }
          frame #9 {
          }
          frame #10 {
          }
          frame #11 {
          }
          frame #12 {
          }
          frame #13 {
          }
          frame #14 {
          }
          frame #15 {
          }
          frame #16 {
          }
          frame #17 {
          }
          frame #18 {
          }
          frame #19 {
          }
          frame #20 {
          }
          frame #21 {
          }
          frame #22 {
          }
          frame #23 {
          }
          frame #24 {
          }
          frame #25 {
          }
          frame #26 {
          }
          frame #27 {
          }
          frame #28 {
          }
          frame #29 {
          }
          frame #30 {
          }
          frame #31 {
          }
          frame #32 {
          }
          frame #33 {
          }
          frame #34 {
          }
        }
        n10 = event shown="[83] \"TestConfiguration\": Shortcut Menu Selection (User)" {
          selector: _ -> [_ _ _ _ _ _ _ _ _ _ _ _ _ _ _ _ _ _ _ _ _ _ _ _ _ _ _ _ _ _ _ _ _ _ _ _ _ _ _ _ _ _ _ _ _ _ _ _ _ _ _ _ _ _ _ _ _ _ _ _ _ _ _ _ _ _ _ _ _ _ _ _ _ _ _ _ _ _ _ _ _ _ _ _ _ _ _ _ _ _ _ _ _ _ _ _ _ _ _ _ _ _ _ _ _ _ _ _ _]
          dyn-events: _ -> [_ _ _ _ _ _ _ _ _ _ _ _ _ _ _ _ _ _ _ _ _ _ _ _ _ _ _ _ _ _ _ _ _ _ _ _ _ _ _ _ _ _ _ _ _ _ _ _ _ _ _ _ _ _ _ _ _ _ _ _ _ _ _ _ _ _ _ _ _ _ _ _ _ _ _ _ _ _ _ _ _ _ _ _ _ _ _ _ _ _ _ _ _ _ _ _ _ _ _ _ _ _ _ _ _ _ _ _ _]
          timeout: 250 ("millisecond multiple") -> [_ _ _ _ _ _ _ _ _ _ _ _ _ _ _ _ _ _ _ _ _ _ _ _ _ _ _ _ _ _ _ _ _ _ _ _ _ _ _ _ _ _ _ _ _ _ _ _ _ _ _ _ _ _ _ _ _ _ _ _ _ _ _ _ _ _ _ _ _ _ _ _ _ _ _ _ _ _ _ _ _ _ _ _ _ _ _ _ _ _ _ _ _ _ _ _ _ _ _ _ _ _ _ _ _ _ _ _ _]
          tunnel: w58 -> [w63 w65 w72 w85 w94 w99 w104 w105 w110 w114 w123 w127 w130 w133 w136 w141 w153 w219 w220 w226 w229 w233 w255 w259 w260 w270 w273 w307 w315 w318 w324 w327 w330 w340 w345 w380 w382 w390 w400 w415 w418 w430 w436 w440 w444 w448 w451 w455 w468 w473 w476 w480 w483 w486 w489 w493 w503 w507 w512 w515 w519 w524 w528 w533 w536 w539 w543 w546 w549 w571 w575 w586 w589 w592 w596 w599 w602 w606 w609 w615 w628 w631 w636 w644 w648 w653 w660 w664 w668 w672 w676 w681 w685 w689 w693 w704 w710 w724 w733 w739 w752 w755 w758 w761 w764 w765 w768 w775 w779]
          tunnel: [w62 w66 w70 w74 w92 w97 w103 w105 w109 w112 w120 w125 w128 w131 w137 w139 w152 w217 w221 w224 w227 w232 w256 w257 w261 w268 w271 w304 w314 w317 w322 w325 w328 w333 w343 w379 w384 w388 w402 w414 w416 w425 w435 w438 w443 w446 w449 w453 w467 w471 w475 w477 w482 w484 w490 w494 w497 w508 w510 w516 w518 w523 w529 w532 w534 w538 w542 w544 w548 w569 w572 w584 w587 w591 w595 w598 w601 w605 w607 w611 w622 w632 w635 w640 w649 w652 w655 w661 w666 w671 w673 w678 w683 w687 w692 w701 w705 w718 w727 w738 w751 w753 w757 w759 w763 w765 w769 w770 w778] -> w56
          tunnel: w53 -> [w61 w64 w71 w82 w93 w98 w102 _ _ _ _ w126 w129 w132 w134 w138 w151 w218 w222 _ w228 _ _ w258 w262 w269 w272 _ w313 w316 w323 w326 w329 w341 w344 w378 w381 _ w399 _ w417 w429 _ _ _ _ w450 _ w469 w472 w474 w479 w481 w485 _ _ _ w505 _ _ _ _ _ w531 w535 w537 w540 w545 w547 w570 w573 w585 w588 w590 _ w597 w600 w604 w608 _ _ _ w634 w643 w650 w651 _ _ _ _ w677 _ _ _ w691 _ w707 w723 w732 w737 w750 w754 w756 w760 w762 _ w767 w774 w777]
          tunnel: w52 -> [_ _ _ _ _ _ _ _ _ _ _ _ _ _ _ _ _ _ _ _ _ _ _ _ _ _ _ _ _ _ _ _ _ _ _ _ _ _ _ _ _ _ _ _ _ _ _ _ _ _ _ _ _ _ _ _ _ _ _ _ _ _ _ _ _ _ _ _ _ _ _ _ _ _ _ _ _ _ _ _ _ _ _ _ _ _ _ _ _ _ _ _ _ _ _ _ _ _ _ _ _ _ _ _ _ _ _ w772 _]
          event "EmergencyStop.LOAD": Value Change {
            n11 = event-data() -> ()  [unwired: 1 in, 1 out]
            n12 = call "ExecEng_EmergencyStip_Sequence_LOAD.vi"("error in (no error)"=w63, "VI Server.RefsCluster"=w61) -> ("error out"=w62:errorcluster)  [unwired: 8 in, 1 out]
          }
          event "EmergencyStop.SAVE": Value Change {
            n13 = event-data() -> ()  [unwired: 1 in, 1 out]
            n14 = call "ExecEng_EmergencyStip_Sequence_SAVE.vi"("error in (no error)"=w65, "VI Server.RefsCluster"=w64) -> ("error out"=w66:errorcluster)  [unwired: 9 in]
          }
          event "EmergencyStop.Sequence": Shortcut Menu Selection (User) {
            n15 = event-data() -> ()  [unwired: 1 in, 2 out]
            n16 = call-poly "VI Server_SetControl.vi"("Data"=string[] [] ("EmergencyStop.Sequence 2"), "Control.Label"="EmergencyStop.Sequence", "error in"=w72, "SingleInstance"=TRUE, "VI Server.RefsCluster"=w71) -> ("error out"=w70:errorcluster)  [unwired: 4 in, 2 out]
          }
          event "EmergencyStop.TEST", "EmergencyStop": Value Change {
            n17 = event-data() -> ()  [unwired: 1 in, 1 out]
            n18 = call "ExEng_Accessor_TestCase_Execution_ABORT_Ref.vi"() -> ("TestCase.Execution.ABORT"=w86:refnum<notifier>)  [unwired: 6 in]
            n19 = Send Notification(notification=TRUE, notifier=w86, error in (no error)=w85) -> (error out=w83:errorcluster)  [unwired: 1 out]
            n20 = call-poly "VI Server_GetControl_Value_Ref.vi"("DataType"=string[] [] ("EmergencyStop.Sequence 2"), "Control.Label"="EmergencyStop.Sequence", "error in"=w83, "SingleInstance"=TRUE, "VI Server.RefsCluster"=w82) -> ("error out"=w78:errorcluster, "Value"=w73:string[])  [unwired: 3 in, 2 out]
            n21 = call "ExEng_Accessor_UDP_Instrument_Instruction_Ref.vi"() -> ("UDP.Instrument.Instruction"=w76:refnum<queue>)  [unwired: 6 in]
            n22 = Flush Queue(queue=w76, error in (no error)=w78) -> (queue out=w75:refnum<queue>, error out=w77:errorcluster)  [unwired: 1 out]
            n23 = for {
              tunnel: w75 -> [w89]
              tunnel: w77 -> [w90]
              tunnel: [w88] -> w74
              tunnel: w73 -> [w87] mode=indexing
              stop <- w88 stop-if-true
              n24 = Enqueue Element(queue=w89, element=w87, error in (no error)=w90) -> (error out=w88:errorcluster)  [unwired: 1 in, 2 out]
            }
          }
          event "Fixture.Slot1", "Fixture.Slot2", "Fixture.Slot3", "Fixture.Slot4", "Fixture.Slot5", "Fixture.Slot6", "Fixture.Slot7", "Fixture.Slot8": Value Change {
            n25 = event-data() -> ()  [unwired: 1 in, 1 out]
            n26 = call "ExecEng_FixtureMgt_SlotsSelector_Init.vi"("CheckReportTemplatePresence"=TRUE, "error in (no error)"=w94, "VI Server.RefsCluster"=w93) -> ("error out"=w92:errorcluster)  [unwired: 7 in, 1 out]
          }
          event "Graph1": Plot Attribute Change {
            n27 = event-data() -> ("OldAttrib"=w96:T7, "NewAttrib"=w95:T7)  [unwired: 1 in]
            n28 = call "ExecEng_AI_Graph1_PlotAttribute_ValueChanged.vi"("NewAttrib"=w95, "OldAttrib"=w96, "error in (no error)"=w99, "VI Server Cluster"=w98) -> ("error out"=w97:errorcluster)  [unwired: 7 in]
          }
          event "Graph2": Plot Attribute Change {
            n29 = event-data() -> ("OldAttrib"=w101:T7, "NewAttrib"=w100:T7)  [unwired: 1 in]
            n30 = call "ExecEng_AI_Graph2_PlotAttribute_ValueChanged.vi"("NewAttrib"=w100, "OldAttrib"=w101, "error in (no error)"=w104, "VI Server Cluster"=w102) -> ("error out"=w103:errorcluster)  [unwired: 7 in]
          }
          event "Help": Value Change {
            n31 = event-data() -> ("NewVal"=w106:bool)  [unwired: 1 in]
            n32 = Control Help Window(1:w106) -> ()  [unwired: 1 in]
          }
          event "Help.Enable": Value Change {
            n33 = event-data() -> ("NewVal"=w107:bool)  [unwired: 1 in]
            n34 = call "ExEng_Accessor_DoNotShowHelp_Ref.vi"() -> ("DoNotShowHelp"=w108:refnum<notifier>)  [unwired: 6 in]
            n35 = Send Notification(notification=w107, notifier=w108, error in (no error)=w110) -> (error out=w109:errorcluster)  [unwired: 1 out]
          }
          event "Instr.Responce.Timeout": Value Change {
            n36 = event-data() -> ("NewVal"=w113:u32)  [unwired: 1 in]
            n37 = call "ExEng_Accessor_Instr_Responce_Timeout_Ref.vi"() -> ("InstructionExecution.InstrResponceTimeOut"=w111:refnum<notifier>)  [unwired: 6 in]
            n38 = Send Notification(notification=w113, notifier=w111, error in (no error)=w114) -> (error out=w112:errorcluster)  [unwired: 1 out]
          }
          event "InstrumentLoad.Disable": Value Change {
            n39 = event-data() -> ("NewVal"=w118:bool)  [unwired: 1 in]
            n40 = call "ExEng_Accessor_InstrumentLoad_Disable_Ref.vi"() -> ("InstrumentLoad.Disable"=w122:refnum<notifier>)  [unwired: 6 in]
            n41 = Send Notification(notification=w118, notifier=w122, error in (no error)=w123) -> (error out=w121:errorcluster)  [unwired: 1 out]
            n42 = Select(t=ExcEng_TestCommand."" ("element"), s=w118, f=ExcEng_TestCommand."Settings.P/N" ("element")) -> (s? t:f=w115:T4)
            n43 = call "ExEng_Accessor_Test_Command_Ref.vi"() -> ("Test.Command"=w119:refnum<queue>)  [unwired: 6 in]
            n44 = Enqueue Element(queue=w119, element=w115, error in (no error)=w121) -> (error out=w120:errorcluster)  [unwired: 1 in, 2 out]
          }
          event "Limit.Units": Value Change {
            n45 = event-data() -> ("NewVal"=w124:string)  [unwired: 1 in]
            n46 = call "ExecEng_Limit_Units.vi"("Limit.Units"=w124, "error in (no error)"=w127, "VI Server.RefsCluster"=w126) -> ("error out"=w125:errorcluster)  [unwired: 8 in]
          }
          event "Limits.Remove": Value Change {
            n47 = event-data() -> ()  [unwired: 1 in, 1 out]
            n48 = call "ExEng_Limits_REMOVE.vi"("error in"=w130, "VI Server.RefsCluster"=w129) -> ("error out"=w128:errorcluster)  [unwired: 8 in, 1 out]
          }
          event "Limits.SAVE": Value Change {
            n49 = event-data() -> ()  [unwired: 1 in, 1 out]
            n50 = call "ExEng_Limits_SAVE.vi"("error in"=w133, "VI Server.RefsCluster"=w132) -> ("error out"=w131:errorcluster)  [unwired: 8 in, 1 out]
          }
          event "Limits.Table": Double Click {
            n51 = event-data() -> ("CtlRef"=w135:refnum<vi>)  [unwired: 1 in]
            n52 = call "ExecEng_LImitsTable_UpdateLimits.vi"("MulticolumnListbox in"=w135, "error in (no error)"=w136, "VI Server.RefsCluster"=w134) -> ("error out"=w137:errorcluster)  [unwired: 8 in]
          }
          event "Limits.Table": Shortcut Menu Selection (User) {
            n53 = event-data() -> ("ItemTag"=w140:string)  [unwired: 1 in]
            n54 = case shown="\"Clear Table\", Default" w140 {
              tunnel: w141 -> [w147 w150]
              tunnel: [w146 w148] -> w139
              tunnel: w138 -> [w145 w149]
              frame "Clear Table", Default {
                n55 = call "VI Server_M_ClmnListBox_ItemNames_SET.vi"("Item Names"=string[][] [], "Label"="Limits.Table", "error in"=w147, "SingleInstance"=TRUE, "VI Server.RefsCluster"=w145) -> ("error out"=w146:errorcluster)  [unwired: 4 in, 2 out]
              }
              frame "Refresh" {
                n56 = call "ExecEng_Refresh Limits Table.vi"("error in (no error)"=w150, "VI Server.RefsCluster.OUT"=w149) -> ("error out"=w148:errorcluster)  [unwired: 9 in]
              }
            }
          }
          event "LimitsIndex": Shortcut Menu Selection (User) {
            n57 = event-data() -> ("ItemTag"=w154:string)  [unwired: 1 in]
            n58 = case shown="\"PATH\"" w154 {
              selector: w154 -> [_ _ w169 _ _ _ _ _]
              tunnel: w153 -> [w155 w167 w171 w184 w196 w208 w210 w214]
              tunnel: [w155 w161 w172 w175 w194 w199 w211 w212] -> w152
              tunnel: w151 -> [_ w159 w170 w183 w195 w207 w209 w213]
              frame "", Default {
              }
              frame "Get Numbers" {
                n59 = call "ExEng_Accessor_UUT_LimitsFile_Ref.vi"() -> ("UUT.LimitsFile"=w168:refnum<notifier>)  [unwired: 6 in]
                n60 = Get Notifier Status(notifier=w168, error in (no error)=w167) -> (current notification=w165:path, error out=w166:errorcluster)  [unwired: 3 out]
                n61 = call "Configuration_GetSectionNames.vi"("Close File"=TRUE, "error in (no error)"=w166, "Configuration.File.Path"=w165) -> ("error out"=w162:errorcluster, "section names"=w164:string[])  [unwired: 5 in, 2 out]
                n62 = Decimal String To Number(string=w164, default (0L)=u16 0 ("default (0 I32)")) -> (number=w158:u16[])  [unwired: 1 in, 1 out]
                n63 = call-poly "VI Server_SetControl.vi"("Data"=w158, "Control.Label"="Limits.List", "error in"=w162, "SingleInstance"=TRUE, "VI Server.RefsCluster"=w159) -> ("error out"=w161:errorcluster)  [unwired: 4 in, 2 out]
              }
              frame "Find" {
                n64 = call "ExecEng_Limit_CheckForConflicts.vi"("ItemTag"=w169, "error in (no error)"=w171, "VI Server.RefsCluster"=w170) -> ("error out"=w172:errorcluster)  [unwired: 8 in]
              }
              frame "STR" {
                w177 = TRUE ("Visible/Unvisible")
                w178 = FALSE ("Visible/Unvisible")
                n65 = call "VI Server_VisibleGroupOfControls.vi"("Defer FP Updating? (T)"=w178, "Visible/Unvisible"=w178, "Labels.Array"=string[] ["Limit.Hi", "Limit.Lo", "Limit.Units", "Limit.PicturePath"], "error in"=w184, "VI Server Cluster"=w183) -> ("error out"=w182:errorcluster, "VI Server Cluster.DUP"=w180:T3)  [unwired: 3 in, 2 out]
                n66 = call "VI Server_VisibleGroupOfControls.vi"("Defer FP Updating? (T)"=w177, "Visible/Unvisible"=w177, "Labels.Array"=string[] ["Limit.Message"], "error in"=w182, "VI Server Cluster"=w180) -> ("error out"=w176:errorcluster)  [unwired: 3 in, 3 out]
                n67 = call "ExEng_Accessor_Limits_Type_Ref.vi"() -> ("Limits.Type"=w174:refnum<notifier>)  [unwired: 6 in]
                n68 = Send Notification(notification=ExecEng_LimitsType."STR", notifier=w174, error in (no error)=w176) -> (error out=w175:errorcluster)  [unwired: 1 out]
              }
              frame "PATH" {
                w189 = TRUE ("Visible/Unvisible")
                w190 = FALSE ("Visible/Unvisible")
                n69 = call "VI Server_VisibleGroupOfControls.vi"("Defer FP Updating? (T)"=w190, "Visible/Unvisible"=w190, "Labels.Array"=string[] ["Limit.Hi", "Limit.Lo", "Limit.Units"], "error in"=w196, "VI Server Cluster"=w195) -> ("error out"=w188:errorcluster, "VI Server Cluster.DUP"=w192:T3)  [unwired: 3 in, 2 out]
                n70 = call "ExEng_Accessor_Limits_Type_Ref.vi"() -> ("Limits.Type"=w186:refnum<notifier>)  [unwired: 6 in]
                n71 = Send Notification(notification=ExecEng_LimitsType."PATH", notifier=w186, error in (no error)=w188) -> (error out=w187:errorcluster)  [unwired: 1 out]
                n72 = call "VI Server_VisibleGroupOfControls.vi"("Defer FP Updating? (T)"=w189, "Visible/Unvisible"=w189, "Labels.Array"=string[] ["Limit.Message", "Limit.PicturePath"], "error in"=w187, "VI Server Cluster"=w192) -> ("error out"=w194:errorcluster)  [unwired: 3 in, 3 out]
              }
              frame "DBL" {
                w201 = FALSE ("Visible/Unvisible")
                w202 = TRUE ("Visible/Unvisible")
                n73 = call "VI Server_VisibleGroupOfControls.vi"("Defer FP Updating? (T)"=w202, "Visible/Unvisible"=w202, "Labels.Array"=string[] ["Limit.Hi", "Limit.Lo", "Limit.Units"], "error in"=w208, "VI Server Cluster"=w207) -> ("error out"=w206:errorcluster, "VI Server Cluster.DUP"=w204:T3)  [unwired: 3 in, 2 out]
                n74 = call "VI Server_VisibleGroupOfControls.vi"("Defer FP Updating? (T)"=w201, "Visible/Unvisible"=w201, "Labels.Array"=string[] ["Limit.Message", "Limit.PicturePath"], "error in"=w206, "VI Server Cluster"=w204) -> ("error out"=w200:errorcluster)  [unwired: 3 in, 3 out]
                n75 = call "ExEng_Accessor_Limits_Type_Ref.vi"() -> ("Limits.Type"=w198:refnum<notifier>)  [unwired: 6 in]
                n76 = Send Notification(notification=ExecEng_LimitsType."DBL", notifier=w198, error in (no error)=w200) -> (error out=w199:errorcluster)  [unwired: 1 out]
              }
              frame "Sort Limits File" {
                n77 = call "ExecEng_SortLimitsFile.vi"("error in (no error)"=w210, "VI Server.RefsCluster.OUT"=w209) -> ("error out"=w211:errorcluster)  [unwired: 9 in]
              }
              frame "Open Limits File" {
                n78 = call "ExecEng_Open Limits File.vi"("error in (no error)"=w214, "VI Server.RefsCluster.OUT"=w213) -> ("error out"=w212:errorcluster)  [unwired: 9 in]
              }
            }
          }
          event "LimitsIndex": Value Change {
            n79 = event-data() -> ()  [unwired: 1 in, 1 out]
            n80 = call "ExEng_TestCaseConfig_LimitsEditor_LimitsIndexValueChanged.vi"("DisplayLimitAssociation"=TRUE ("DisplayLimitAssociaation"), "ResetControls'Visibility"=TRUE, "error in"=w219, "VI Server.RefsCluster"=w218) -> ("error out"=w217:errorcluster)  [unwired: 6 in, 1 out]
          }
          event "Mem.RST": Value Change {
            n81 = event-data() -> ()  [unwired: 1 in, 1 out]
            n82 = call "ExecEng_Function_Clear_Memory_Num.vi"("error in (no error)"=w220, "VI Server Custer"=w222) -> ("error out"=w221:errorcluster)  [unwired: 8 in, 1 out]
          }
          event "MEM.RST.AtTestStart": Value Change {
            n83 = event-data() -> ("NewVal"=w223:bool)  [unwired: 1 in]
            n84 = call "ExEng_Accessor_MEM_RST_AtTestStart_Ref.vi"() -> ("MEM.RST.AtTestStart"=w225:refnum<notifier>)  [unwired: 6 in]
            n85 = Send Notification(notification=w223, notifier=w225, error in (no error)=w226) -> (error out=w224:errorcluster)  [unwired: 1 out]
          }
          event "Mem.Str.RST": Value Change {
            n86 = event-data() -> ()  [unwired: 1 in, 1 out]
            n87 = call "ExecEng_Function_Clear_MemoryStr.vi"("error in (no error)"=w229, "VI Server Custer"=w228) -> ("error out"=w227:errorcluster)  [unwired: 8 in, 1 out]
          }
          event "Mem1", "Mem10", "Mem11", "Mem12", "Mem13", "Mem14", "Mem15", "Mem16", "Mem100", "Mem101", "Mem102", "Mem103", "Mem104", "Mem105", "Mem106", "Mem107", "Mem108", "Mem109", "Mem110", "Mem111", "Mem112", "Mem17", "Mem18", "Mem19", "Mem113", "Mem114", "Mem115", "Mem116", "Mem117", "Mem118", "Mem119", "Mem120", "Mem121", "Mem122", "Mem123", "Mem124", "Mem125", "Mem126", "Mem127", "Mem128", "Mem129", "Mem130", "Mem131", "Mem132", "Mem133", "Mem134", "Mem135", "Mem136", "Mem137", "Mem138", "Mem139", "Mem140", "Mem141", "Mem142", "Mem143", "Mem144", "Mem145", "Mem146", "Mem147", "Mem148", "Mem149", "Mem150", "Mem151", "Mem152", "Mem153", "Mem154", "Mem155", "Mem156", "Mem157", "Mem158", "Mem159", "Mem160", "Mem161", "Mem162", "Mem163", "Mem164", "Mem165", "Mem166", "Mem167", "Mem168", "Mem169", "Mem170", "Mem171", "Mem172", "Mem173", "Mem174", "Mem175", "Mem176", "Mem177", "Mem178", "Mem179", "Mem180", "Mem181", "Mem182", "Mem183", "Mem184", "Mem185", "Mem186", "Mem187", "Mem188", "Mem189", "Mem190", "Mem191", "Mem192", "Mem2", "Mem20", "Mem21", "Mem22", "Mem23", "Mem24", "Mem25", "Mem26", "Mem27", "Mem28", "Mem29", "Mem3", "Mem30", "Mem31", "Mem32", "Mem33", "Mem34", "Mem35", "Mem36", "Mem37", "Mem38", "Mem39", "Mem4", "Mem40", "Mem41", "Mem42", "Mem43", "Mem44", "Mem45", "Mem46", "Mem47", "Mem48", "Mem49", "Mem5", "Mem50", "Mem51", "Mem52", "Mem53", "Mem54", "Mem55", "Mem56", "Mem57", "Mem58", "Mem59", "Mem6", "Mem60", "Mem61", "Mem62", "Mem63", "Mem64", "Mem65", "Mem66", "Mem67", "Mem68", "Mem69", "Mem7", "Mem70", "Mem71", "Mem72", "Mem73", "Mem74", "Mem75", "Mem76", "Mem77", "Mem78", "Mem79", "Mem8", "Mem80", "Mem81", "Mem82", "Mem83", "Mem84", "Mem85", "Mem86", "Mem87", "Mem88", "Mem89", "Mem9", "Mem97", "Mem98", "Mem99", "Mem90", "Mem91", "Mem92", "Mem93", "Mem94", "Mem95", "Mem96", "Mem193", "Mem194", "Mem195", "Mem196", "Mem197", "Mem198", "Mem199", "Mem288", "Mem287", "Mem286", "Mem285", "Mem284", "Mem283", "Mem282", "Mem281", "Mem280", "Mem279", "Mem278", "Mem277", "Mem276", "Mem275", "Mem274", "Mem273", "Mem272", "Mem271", "Mem270", "Mem269", "Mem268", "Mem267", "Mem266", "Mem265", "Mem264", "Mem263", "Mem262", "Mem261", "Mem260", "Mem259", "Mem258", "Mem257", "Mem256", "Mem255", "Mem254", "Mem253", "Mem252", "Mem251", "Mem250", "Mem249", "Mem248", "Mem247", "Mem246", "Mem245", "Mem244", "Mem243", "Mem242", "Mem241", "Mem240", "Mem239", "Mem238", "Mem237", "Mem236", "Mem235", "Mem234", "Mem233", "Mem232", "Mem231", "Mem230", "Mem229", "Mem228", "Mem227", "Mem226", "Mem225", "Mem224", "Mem223", "Mem222", "Mem221", "Mem220", "Mem219", "Mem218", "Mem217", "Mem216", "Mem215", "Mem214", "Mem213", "Mem212", "Mem211", "Mem210", "Mem209", "Mem299", "Mem298", "Mem297", "Mem296", "Mem295", "Mem294", "Mem293", "Mem292", "Mem291", "Mem290", "Mem289", "Mem384", "Mem208", "Mem207", "Mem206", "Mem205", "Mem204", "Mem202", "Mem201", "Mem200", "Mem383", "Mem382", "Mem381", "Mem380", "Mem379", "Mem378", "Mem377", "Mem376", "Mem375", "Mem374", "Mem373", "Mem372", "Mem371", "Mem370", "Mem369", "Mem368", "Mem367", "Mem366", "Mem365", "Mem364", "Mem363", "Mem362", "Mem361", "Mem360", "Mem359", "Mem358", "Mem357", "Mem356", "Mem355", "Mem354", "Mem353", "Mem352", "Mem351", "Mem350", "Mem349", "Mem348", "Mem347", "Mem346", "Mem345", "Mem344", "Mem343", "Mem341", "Mem340", "Mem339", "Mem338", "Mem337", "Mem336", "Mem335", "Mem334", "Mem333", "Mem332", "Mem331", "Mem330", "Mem329", "Mem328", "Mem327", "Mem326", "Mem325", "Mem324", "Mem323", "Mem322", "Mem321", "Mem320", "Mem319", "Mem318", "Mem317", "Mem316", "Mem315", "Mem314", "Mem313", "Mem312", "Mem311", "Mem310", "Mem309", "Mem308", "Mem307", "Mem305", "Mem304", "Mem303", "Mem302", "Mem301", "Mem300": Shortcut Menu Selection (User) {
            n88 = event-data() -> ("CtlRef"=w231:refnum<vi>, "ItemTag"=w230:string)  [unwired: 1 in]
            n89 = case shown="\"Format String\"" w230 {
              tunnel: w233 -> [w234 w237 w242 w247 w252]
              tunnel: [w234 w236 w240 w245 w251] -> w232
              tunnel: w231 -> [_ w235 w243 w249 w253]
              frame "False", Default {
              }
              frame "Format String" {
                n90 = call "ExecEng_Message_MemoryCtl_FormatString.vi"("CtlRef"=w235, "error in"=w237) -> ("error out"=w236:errorcluster)  [unwired: 9 in]
              }
              frame "Copy Format String" {
                n91 = property on="Property Node" class="DigNum (strict)"(reference=w243, error in=w242) -> (error out=w241:errorcluster, "FormatString"=w238:string)  [unwired: 1 out]
                n92 = call "ExEng_Accessor_Mem_FormatStr_Ref.vi"() -> ("Mem.FormatStr"=w239:refnum<notifier>)  [unwired: 6 in]
                n93 = Send Notification(notification=w238, notifier=w239, error in (no error)=w241) -> (error out=w240:errorcluster)  [unwired: 1 out]
              }
              frame "Paste Format String" {
                n94 = call "ExEng_Accessor_Mem_FormatStr_Ref.vi"() -> ("Mem.FormatStr"=w248:refnum<notifier>)  [unwired: 6 in]
                n95 = Get Notifier Status(notifier=w248, error in (no error)=w247) -> (current notification=w244:string, error out=w246:errorcluster)  [unwired: 3 out]
                n96 = property on="Property Node" class="DigNum (strict)"(reference=w249, error in=w246, "FormatString"=w244) -> (error out=w245:errorcluster)  [unwired: 1 out]
              }
              frame "Stop Blinking" {
                n97 = property on="Property Node" class="DigNum (strict)"(reference=w253, error in=w252, "Blinking"=FALSE) -> (error out=w251:errorcluster)  [unwired: 1 out]
              }
            }
          }
          event "Mem1", "Mem2", "Mem3", "Mem4", "Mem5", "Mem6", "Mem7", "Mem8", "Mem9", "Mem10", "Mem11", "Mem12", "Mem13", "Mem14", "Mem15", "Mem16", "Mem97", "Mem98", "Mem99", "Mem100", "Mem101", "Mem102", "Mem103", "Mem104", "Mem105", "Mem106", "Mem107", "Mem108", "Mem109", "Mem110", "Mem111", "Mem112", "Mem17", "Mem18", "Mem19", "Mem20", "Mem21", "Mem22", "Mem23", "Mem24", "Mem25", "Mem26", "Mem27", "Mem28", "Mem29", "Mem30", "Mem31", "Mem32", "Mem113", "Mem114", "Mem115", "Mem116", "Mem117", "Mem118", "Mem119", "Mem120", "Mem121", "Mem122", "Mem123", "Mem124", "Mem125", "Mem126", "Mem127", "Mem128", "Mem33", "Mem34", "Mem35", "Mem36", "Mem37", "Mem38", "Mem39", "Mem40", "Mem41", "Mem42", "Mem43", "Mem44", "Mem45", "Mem46", "Mem47", "Mem48", "Mem129", "Mem130", "Mem131", "Mem132", "Mem133", "Mem134", "Mem135", "Mem136", "Mem137", "Mem138", "Mem139", "Mem140", "Mem141", "Mem142", "Mem143", "Mem144", "Mem49", "Mem50", "Mem51", "Mem52", "Mem53", "Mem54", "Mem55", "Mem56", "Mem57", "Mem58", "Mem60", "Mem59", "Mem61", "Mem62", "Mem63", "Mem64", "Mem145", "Mem146", "Mem147", "Mem148", "Mem149", "Mem150", "Mem151", "Mem152", "Mem153", "Mem154", "Mem155", "Mem156", "Mem157", "Mem158", "Mem159", "Mem160", "Mem65", "Mem66", "Mem67", "Mem68", "Mem69", "Mem70", "Mem71", "Mem72", "Mem73", "Mem74", "Mem75", "Mem76", "Mem77", "Mem78", "Mem79", "Mem80", "Mem161", "Mem162", "Mem163", "Mem164", "Mem165", "Mem166", "Mem167", "Mem168", "Mem169", "Mem170", "Mem171", "Mem172", "Mem173", "Mem174", "Mem175", "Mem176", "Mem81", "Mem82", "Mem83", "Mem84", "Mem85", "Mem86", "Mem87", "Mem88", "Mem89", "Mem90", "Mem91", "Mem92", "Mem93", "Mem94", "Mem95", "Mem96", "Mem177", "Mem178", "Mem179", "Mem180", "Mem181", "Mem182", "Mem183", "Mem184", "Mem185", "Mem186", "Mem187", "Mem188", "Mem189", "Mem190", "Mem191", "Mem192", "Mem199", "Mem198", "Mem197", "Mem196", "Mem195", "Mem194", "Mem193", "Mem203", "Mem288", "Mem287", "Mem286", "Mem285", "Mem284", "Mem283", "Mem282", "Mem281", "Mem280", "Mem279", "Mem278", "Mem277", "Mem276", "Mem275", "Mem274", "Mem273", "Mem272", "Mem271", "Mem270", "Mem269", "Mem268", "Mem267", "Mem266", "Mem265", "Mem264", "Mem263", "Mem262", "Mem261", "Mem260", "Mem259", "Mem258", "Mem257", "Mem256", "Mem255", "Mem254", "Mem253", "Mem252", "Mem251", "Mem250", "Mem249", "Mem248", "Mem247", "Mem246", "Mem245", "Mem244", "Mem243", "Mem242", "Mem241", "Mem240", "Mem239", "Mem237", "Mem236", "Mem235", "Mem234", "Mem233", "Mem232", "Mem231", "Mem230", "Mem229", "Mem228", "Mem227", "Mem226", "Mem225", "Mem224", "Mem223", "Mem222", "Mem221", "Mem220", "Mem219", "Mem218", "Mem217", "Mem216", "Mem215", "Mem214", "Mem213", "Mem212", "Mem211", "Mem210", "Mem209", "Mem299", "Mem298", "Mem297", "Mem296", "Mem295", "Mem294", "Mem293", "Mem292", "Mem291", "Mem290", "Mem289", "Mem384", "Mem208", "Mem207", "Mem206", "Mem205", "Mem204", "Mem202", "Mem201", "Mem200", "Mem383", "Mem382", "Mem381", "Mem380", "Mem379", "Mem378", "Mem377", "Mem376", "Mem375", "Mem374", "Mem373", "Mem372", "Mem371", "Mem370", "Mem369", "Mem368", "Mem367", "Mem366", "Mem365", "Mem364", "Mem363", "Mem362", "Mem361", "Mem360", "Mem359", "Mem358", "Mem357", "Mem356", "Mem355", "Mem354", "Mem353", "Mem352", "Mem351", "Mem350", "Mem349", "Mem348", "Mem347", "Mem346", "Mem345", "Mem344", "Mem343", "Mem342", "Mem341", "Mem340", "Mem339", "Mem338", "Mem337", "Mem336", "Mem335", "Mem334", "Mem333", "Mem332", "Mem331", "Mem330", "Mem329", "Mem328", "Mem327", "Mem326", "Mem325", "Mem324", "Mem323", "Mem322", "Mem321", "Mem320", "Mem319", "Mem318", "Mem317", "Mem316", "Mem315", "Mem314", "Mem313", "Mem312", "Mem311", "Mem310", "Mem309", "Mem308", "Mem307", "Mem306", "Mem305", "Mem304", "Mem303", "Mem302", "Mem301", "Mem300": Shortcut Menu Activation? {
            n98 = event-data() -> ("MenuRef"=w254:refnum<k9>)  [unwired: 1 in]
            n99 = call "ExecEng_Memory_ActivateUserShortCutMenu.vi"("Menu in"=w254, "error in (no error)"=w255) -> ("error out"=w256:errorcluster)  [unwired: 9 in]
            n100 = event-data ("Event Filter Node")() -> ()  [unwired: 2 in, 1 out]
          }
          event "Num.Memory.LOAD": Value Change {
            n101 = event-data() -> ()  [unwired: 1 in, 1 out]
            n102 = call "ExecEng_NumMEmory_LOAD.vi"("error in (no error)"=w259, "VI Server.RefsCluster"=w258) -> ("error out"=w257:errorcluster)  [unwired: 9 in]
          }
          event "Num.Memory.SAVE": Value Change {
            n103 = event-data() -> ()  [unwired: 1 in, 1 out]
            n104 = call "ExecEng_NumMEmory_SAVE.vi"("error in (no error)"=w260, "VI Server.RefsCluster"=w262) -> ("error out"=w261:errorcluster)  [unwired: 8 in, 1 out]
          }
          event "NumMem.FailedUpdates": Double Click {
            n105 = event-data() -> ("Row"=w263:i32)  [unwired: 1 in]
            n106 = call "VI Server_M_ClmnListBox_1orMoreSelection_ItemNames_GET.vi"("Label"="NumMem.FailedUpdates", "error in"=w270, "SingleInstance"=TRUE, "VI Server.RefsCluster"=w269) -> ("error out"=w265:errorcluster, "Multicolumn Listbox.Ref"=w264:refnum<vi>)  [unwired: 1 in, 5 out]
            n107 = property on="Property Node" class="MCListbox (strict)"(reference=w264, error in=w265, "Value"=w263) -> (error out=w268:errorcluster)  [unwired: 1 out]
          }
          event "NumMem.FailedUpdates": Shortcut Menu Selection (User) {
            n108 = event-data() -> ("ItemTag"=w274:string)  [unwired: 1 in]
            n109 = case shown="\"Find\"" w274 {
              tunnel: w273 -> [w275 w284 w292 w303]
              tunnel: w272 -> [_ w283 w291 w302]
              tunnel: [w275 w277 w286 w295] -> w271
              frame "False", Default {
              }
              frame "Clear Table" {
                n110 = call "VI Server_M_ClmnListBox_ItemNames_SET.vi"("Item Names"=string[][] [], "Label"="NumMem.FailedUpdates", "error in"=w284, "SingleInstance"=TRUE, "VI Server.RefsCluster"=w283) -> ("error out"=w279:errorcluster, "Multicolumn Listbox.Ref"=w278:refnum<vi>)  [unwired: 4 in, 1 out]
                n111 = property on="Property Node" class="MCListbox (strict)"(reference=w278, error in=w279, "Value"=0) -> (error out=w277:errorcluster)  [unwired: 1 out]
              }
              frame "Clear Selection" {
                n112 = call "VI Server_M_ClmnListBox_1orMoreSelection_ItemNames_GET.vi"("Label"="NumMem.FailedUpdates", "error in"=w292, "SingleInstance"=TRUE, "VI Server.RefsCluster"=w291) -> ("error out"=w288:errorcluster, "Multicolumn Listbox.Ref"=w287:refnum<vi>)  [unwired: 1 in, 5 out]
                n113 = property on="Property Node" class="MCListbox (strict)"(reference=w287, error in=w288, "Value"=0) -> (error out=w286:errorcluster)  [unwired: 1 out]
              }
              frame "Find" {
                w293 = TRUE ("SingleInstance")
                n114 = call "VI Server_M_ClmnListBox_SelectedCell_GET.vi"("Label"="NumMem.FailedUpdates", "error in"=w303, "SingleInstance"=w293, "VI Server.RefsCluster"=w302) -> ("error out"=w300:errorcluster, "Cell.String"=w299:string, "VI Server.RefsCluster.DUP"=w298:T3)  [unwired: 4 in, 1 out]
                n115 = call-poly "VI Server_GetControl_Value_Ref.vi"("DataType"=0.0, "Control.Label"=w299, "error in"=w300, "SingleInstance"=w293, "VI Server.RefsCluster"=w298) -> ("error out"=w296:errorcluster, "Control.Ref"=w294:refnum<vi>)  [unwired: 3 in, 2 out]
                n116 = property on="Property Node" class="DigNum (strict)"(reference=w294, error in=w296, "Blinking"=w293) -> (error out=w295:errorcluster)  [unwired: 1 out]
              }
            }
          }
          event "NumMemory.Blinking": Value Change {
            n117 = event-data() -> ("NewVal"=w305:bool)  [unwired: 1 in]
            n118 = call "ExEng_Accessor_NumMemory_Blinking_Ref.vi"() -> ("NumMemory.Blinking"=w306:refnum<notifier>)  [unwired: 6 in]
            n119 = Send Notification(notification=w305, notifier=w306, error in (no error)=w307) -> (error out=w304:errorcluster)  [unwired: 1 out]
          }
          event "Performance.Verification.Enable": Value Change {
            n120 = event-data() -> ("NewVal"=w310:bool)  [unwired: 1 in]
            n121 = Select(t=T2."Enabled" ("Enable/Disable"), s=w310, f=T2."Disabled and Grayed Out") -> (s? t:f=w308:T2)
            n122 = call "VI Server_EnableDisable Group of Controls.vi"("Enable/Disable"=w308, "Labels.Array"=string[] ["Performance.Verification.Pass/Fail", "Performance.Verification.SAVE"], "error in"=w315, "VI Server Cluster"=w313) -> ("error out"=w314:errorcluster)  [unwired: 5 in, 2 out]
          }
          event "Performance.Verification.SAVE": Value Change {
            n123 = event-data() -> ()  [unwired: 1 in, 1 out]
            n124 = call "ExecEng_PerformanceVerification_SAVE.vi"("error in"=w318, "VI Server.RefsCluster"=w316) -> ("error out"=w317:errorcluster)  [unwired: 8 in, 1 out]
          }
          event "Report.PDF.File.Content.Clear": Value Change {
            n125 = event-data() -> ()  [unwired: 1 in, 1 out]
            n126 = call-poly "VI Server_SetControl.vi"("New Value"="" ("Empty String Constant"), "Label"="Report.PDF.File.Content", "error in"=w324, "Single Instance (T)"=TRUE ("SingleInstance"), "VI Server Cluster"=w323) -> ("error out"=w322:errorcluster)  [unwired: 4 in, 2 out]
          }
          event "Report.PDF.File.Read": Value Change {
            n127 = event-data() -> ()  [unwired: 1 in, 1 out]
            n128 = call "ExecEng_Report_PDF_File_Read.vi"("error in (no error)"=w327, "VI Server.RefsCluster"=w326) -> ("error out"=w325:errorcluster)  [unwired: 9 in]
          }
          event "Report.PDF.OpenWithACROBAT": Value Change {
            n129 = event-data() -> ()  [unwired: 1 in, 1 out]
            n130 = call "ExecEng_Report_PDF_File_Open_with_ACROBAT.vi"("error in (no error)"=w330, "VI Server.RefsCluster"=w329) -> ("error out"=w328:errorcluster)  [unwired: 9 in]
          }
          event "Report.Test": Value Change {
            n131 = event-data() -> ()  [unwired: 1 in, 3 out]
            n132 = call "ExEng_Accessor_Test_Report_Skip_Ref.vi"() -> ("Test.Report.Skip"=w339:refnum<notifier>)  [unwired: 6 in]
            n133 = Get Notifier Status(notifier=w339, error in (no error)=w340) -> (notifier out=w336:refnum<notifier>, current notification=w331:bool, error out=w338:errorcluster)  [unwired: 2 out]
            n134 = Send Notification(notification=FALSE, notifier=w336, error in (no error)=w338) -> (notifier out=w332:refnum<notifier>, error out=w337:errorcluster)
            n135 = call "ExecEng_REPORT_MAIN_MultiSlots.vi"("error in"=w337, "VI Server.RefsCluster"=w341) -> ("error out"=w334:errorcluster)  [unwired: 8 in, 1 out]
            n136 = Send Notification(notification=w331, notifier=w332, error in (no error)=w334) -> (error out=w333:errorcluster)  [unwired: 1 out]
          }
          event "SerialNumbers.Array": Shortcut Menu Selection (User) {
            n137 = event-data() -> ("ItemTag"=w342:string)  [unwired: 1 in]
            n138 = case shown="\"Enable\"" w342 {
              tunnel: w345 -> [w346 w355 w374]
              tunnel: w344 -> [_ w357 w375]
              tunnel: [w346 w350 w371] -> w343
              frame "False", Default {
              }
              frame "Enable" {
                n139 = for {
                  tunnel: w357 -> [w366]
                  tunnel: [w367] -> w358
                  tunnel: w355 -> [w365]
                  tunnel: [w363] -> w356
                  tunnel: string[] ["Fixture.Slot1", "Fixture.Slot2", "Fixture.Slot3", "Fixture.Slot4", "Fixture.Slot5", "Fixture.Slot6", "Fixture.Slot7", "Fixture.Slot8"] -> [w362] mode=indexing
                  tunnel: [""] -> w347 mode=indexing if=w360
                  stop <- w363 stop-if-true
                  w364 = FALSE ("SingleInstance")
                  n140 = call-poly "VI Server_GetControl_Value_Ref.vi"("DataType"=w364, "Control.Label"=w362, "error in"=w365, "SingleInstance"=w364, "VI Server.RefsCluster"=w366) -> ("error out"=w363:errorcluster, "Value"=w360:bool, "VI Server.RefsCluster.DUP"=w367:T3)  [unwired: 3 in, 1 out]
                }
                n141 = call-poly "VI Server_GetControl_Value_Ref.vi"("DataType"=string[] [], "Control.Label"="SerialNumbers.Array" ("Label"), "error in"=w356, "SingleInstance"=TRUE, "VI Server.RefsCluster"=w358) -> ("error out"=w351:errorcluster, "Control.Ref"=w349:refnum<vi>)  [unwired: 3 in, 2 out]
                n142 = property on="Property Node" class="Arr (strict)"(reference=w349, error in=w351, "DisabledEnum"=T2."Enabled" ("Disabled"), "Value"=w347) -> (error out=w350:errorcluster)  [unwired: 1 out]
              }
              frame "Disable & Gray Out" {
                w368 = string[] []
                n143 = call-poly "VI Server_GetControl_Value_Ref.vi"("DataType"=w368, "Control.Label"="SerialNumbers.Array" ("Label"), "error in"=w374, "SingleInstance"=TRUE, "VI Server.RefsCluster"=w375) -> ("error out"=w372:errorcluster, "Control.Ref"=w370:refnum<vi>)  [unwired: 3 in, 2 out]
                n144 = property on="Property Node" class="Arr (strict)"(reference=w370, error in=w372, "DisabledEnum"=T2."Disabled and Grayed Out" ("Disabled"), "Value"=w368) -> (error out=w371:errorcluster)  [unwired: 1 out]
              }
            }
          }
          event "Settings.P/N": Shortcut Menu Selection (User) {
            n145 = event-data() -> ("ItemTag"=w377:string)  [unwired: 1 in]
            n146 = call "ExEng_Settings_PartNumbers_UserMenu.vi"("ItemTag"=w377, "error in"=w380, "VI Server.RefsCluster"=w378) -> ("error out"=w379:errorcluster)  [unwired: 7 in, 1 out]
          }
          event "Settings.P/N": Value Change {
            n147 = event-data() -> ()  [unwired: 1 in, 1 out]
            n148 = call "ExEng_Accessor_Test_Command_Ref.vi"() -> ("Test.Command"=w386:refnum<queue>)  [unwired: 6 in]
            n149 = call "ExEng_Settings_Test_PartNumber_Selected.vi"("error in"=w382, "VI Server.RefsCluster"=w381) -> ("error out"=w383:errorcluster)  [unwired: 8 in, 1 out]
            n150 = Enqueue Element(queue=w386, element=ExcEng_TestCommand."Settings.P/N", error in (no error)=w383) -> (error out=w384:errorcluster)  [unwired: 1 in, 2 out]
          }
          event "SimulateTestFailure": Value Change {
            n151 = event-data() -> ()  [unwired: 1 in, 1 out]
            n152 = call "ExEng_Accessor_TestCase_Execute_Pass_Fail_Ref.vi"() -> ("TestCase.Execute.Pass/Fail"=w389:refnum<queue>)  [unwired: 6 in]
            n153 = Enqueue Element(queue=w389, element=FALSE, error in (no error)=w390) -> (error out=w388:errorcluster)  [unwired: 1 in, 2 out]
          }
          event "Test.ABORT", "TestCase.Diagnostics.ABORT", "TestCase.Execute.ABORT": Value Change {
            n154 = event-data() -> ()  [unwired: 1 in, 1 out]
            n155 = call-poly "VI Server_SetControl.vi"("Data"=FALSE, "Control.Label"="Test.ABORT", "error in"=w400, "SingleInstance"=TRUE, "VI Server.RefsCluster"=w399) -> ("error out"=w395:errorcluster, "VI Server.RefsCluster.DUP"=w393:T3)  [unwired: 4 in, 1 out]
            n156 = call "VI Server_Enable_Disable.vi"("Disabled"=T2."Enabled", "Label"="TestCase.SAVE", "error in"=w395, "VI Server Cluster"=w393) -> ("error out"=w394:errorcluster)  [unwired: 5 in, 2 out]
            n157 = call "ExEng_Accessor_TestCase_Execution_ABORT_Ref.vi"() -> ("TestCase.Execution.ABORT"=w410:refnum<notifier>)  [unwired: 6 in]
            n158 = call "ExEng_Accessor_MainVI_Menu_Ref.vi"() -> ("MainVI.MenuRef"=w409:refnum<notifier>)  [unwired: 6 in]
            n159 = Send Notification(notification=TRUE, notifier=w410, error in (no error)=w394) -> (error out=w408:errorcluster)  [unwired: 1 out]
            n160 = Get Notifier Status(notifier=w409, error in (no error)=w408) -> (current notification=w406:refnum<k9>, error out=w407:errorcluster)  [unwired: 3 out]
            n161 = call "Menu ~ForsedCheck_Uncheck Item .vi"("error in (no error)"=w407, "item tag"="Repeat Test", "menubar"=w406) -> ("error out"=w403:errorcluster)  [unwired: 6 in, 2 out]
            n162 = call "ExEng_Accessor_Test_Repeat_Ref.vi"() -> ("Test.Repeat"=w404:refnum<notifier>)  [unwired: 6 in]
            n163 = Send Notification(notification=FALSE, notifier=w404, error in (no error)=w403) -> (error out=w402:errorcluster)  [unwired: 1 out]
          }
          event "Test.Instruments.FP": Value Change {
            n164 = event-data() -> ("NewVal"=w413:bool)  [unwired: 1 in]
            n165 = call "ExEng_Accessor_Test_Instruments_FP_Ref.vi"() -> ("Test.Instruments.FP"=w412:refnum<notifier>)  [unwired: 6 in]
            n166 = Send Notification(notification=w413, notifier=w412, error in (no error)=w415) -> (error out=w414:errorcluster)  [unwired: 1 out]
          }
          event "Test.P/N": Value Change {
            n167 = event-data() -> ()  [unwired: 1 in, 1 out]
            n168 = call "ExEng_Test_PartNumber_Selected.vi"("error in"=w418, "VI Server.RefsCluster"=w417) -> ("error out"=w416:errorcluster)  [unwired: 8 in, 1 out]
          }
          event "Test.Pause": Value Change {
            n169 = event-data() -> ("NewVal"=w422:bool)  [unwired: 1 in]
            n170 = call "VI Server_Enable_Disable.vi"("Disabled"=T2."Enabled", "Label"="TestCase.SAVE", "error in"=w430, "VI Server Cluster"=w429) -> ("error out"=w431:errorcluster, "VI Server Cluster.DUP"=w424:T3)  [unwired: 5 in, 1 out]
            n171 = call "ExEng_Accessor_TestExecution_Pause_Ref.vi"() -> ("Test.Execution.Pause"=w432:refnum<notifier>)  [unwired: 6 in]
            n172 = Send Notification(notification=w422, notifier=w432, error in (no error)=w431) -> (error out=w426:errorcluster)  [unwired: 1 out]
            n173 = Select(t=T2."Enabled" ("Enable/Disable"), s=w422, f=T2."Disabled and Grayed Out") -> (s? t:f=w419:T2)
            n174 = call "VI Server_EnableDisable Group of Controls.vi"("Enable/Disable"=w419, "Labels.Array"=string[] ["TestCase.Execute.Selected", "TestCase.Execute.All"], "error in"=w426, "VI Server Cluster"=w424) -> ("error out"=w425:errorcluster)  [unwired: 5 in, 2 out]
          }
          event "Test.PauseOnFailure": Value Change {
            n175 = event-data() -> ("NewVal"=w434:bool)  [unwired: 1 in]
            n176 = call "ExEng_Accessor_TestCaseExecution_StopOnFailure_Ref.vi"() -> ("TestCaseExecution.PauseOnFailure"=w433:refnum<notifier>)  [unwired: 6 in]
            n177 = Send Notification(notification=w434, notifier=w433, error in (no error)=w436) -> (error out=w435:errorcluster)  [unwired: 1 out]
          }
          event "Test.Repeat.NumberOf": Value Change {
            n178 = event-data() -> ("NewVal"=w437:i32)  [unwired: 1 in]
            n179 = call "ExEng_Accessor_TestRepeat_NumberOf_Ref.vi"() -> ("Test.Repeat.NumberOf"=w439:refnum<notifier>)  [unwired: 6 in]
            n180 = Send Notification(notification=w437, notifier=w439, error in (no error)=w440) -> (error out=w438:errorcluster)  [unwired: 1 out]
          }
          event "Test.Report.Skip": Value Change {
            n181 = event-data() -> ("NewVal"=w442:bool)  [unwired: 1 in]
            n182 = call "ExEng_Accessor_Test_Report_Skip_Ref.vi"() -> ("Test.Report.Skip"=w441:refnum<notifier>)  [unwired: 6 in]
            n183 = Send Notification(notification=w442, notifier=w441, error in (no error)=w444) -> (error out=w443:errorcluster)  [unwired: 1 out]
          }
          event "Test.Results.LogFile.Folder": Value Change {
            n184 = event-data() -> ("NewVal"=w445:path)  [unwired: 1 in]
            n185 = call "ExEng_Accessor_Test_Failure_LogFile_Ref.vi"() -> ("Test.Failure.LogFile"=w447:refnum<notifier>)  [unwired: 6 in]
            n186 = Send Notification(notification=w445, notifier=w447, error in (no error)=w448) -> (error out=w446:errorcluster)  [unwired: 1 out]
          }
          event "Test.Start": Value Change {
            n187 = event-data() -> ()  [unwired: 1 in, 1 out]
            n188 = call "ExecEng_TEST_Start.vi"("error in (no error)"=w451, "VI Server.RefsCluster"=w450) -> ("error out"=w449:errorcluster)  [unwired: 9 in]
          }
          event "Test.StartTime", "Test.EndTime", "Test.Start.DateTime", "Test.End.DateTime": Shortcut Menu Selection (User) {
            n189 = event-data() -> ("CtlRef"=w452:refnum<vi>, "ItemTag"=w454:string)  [unwired: 1 in]
            n190 = case shown="No Error" w455 {
              selector: w455 -> [w458 w465]
              tunnel: w454 -> [w459 _]
              tunnel: [w457 w465] -> w453
              tunnel: w452 -> [w456 _]
              frame No Error {
                n191 = case shown="\"Insert present time\"" w459 {
                  tunnel: w458 -> [w460 w464]
                  tunnel: [w460 w462] -> w457
                  tunnel: w456 -> [_ w463]
                  frame "", Default {
                  }
                  frame "Insert present time" {
                    n192 = call "EecEng_Get_Current_Date_Time.vi"() -> ("Time (mm/dd/yy h:m:s)"=w461:string)  [unwired: 7 in]
                    n193 = property on="Property Node" class="Str"(reference=w463, error in=w464, "Value"=w461) -> (error out=w462:errorcluster)  [unwired: 1 out]
                  }
                }
              }
              frame Error {
              }
            }
          }
          event "Test.Tree": Item Close {
            n194 = event-data() -> ("Tag"=w466:string)  [unwired: 1 in]
            n195 = call "ExecEng_Tree_ItemClose.vi"("Tag"=w466, "error in (no error)"=w468, "VI Server.RefsCluster"=w469) -> ("error out"=w467:errorcluster)  [unwired: 8 in]
          }
          event "Test.Tree": Shortcut Menu Selection (User) {
            n196 = event-data() -> ("ItemTag"=w470:string)  [unwired: 1 in]
            n197 = call "ExecEng_Tree_UserMenu.vi"("ItemTag"=w470, "error in (no error)"=w473, "VI Server.RefsCluster"=w472) -> ("error out"=w471:errorcluster)  [unwired: 8 in]
          }
          event "Test.Tree": Value Change {
            n198 = event-data() -> ()  [unwired: 1 in, 1 out]
            n199 = call "ExecEng_Test_Tree_ValueChanged.vi"("error in (no error)"=w476, "VI Server.RefsCluster"=w474) -> ("error out"=w475:errorcluster)  [unwired: 9 in]
          }
          event "TestCase": Shortcut Menu Selection (User) {
            n200 = event-data() -> ("ItemTag"=w478:string)  [unwired: 1 in]
            n201 = call "ExEng_Settings_TestCase_UserMenu.vi"("ItemTag"=w478, "error in"=w480, "VI Server.RefsCluster"=w479) -> ("error out"=w477:errorcluster)  [unwired: 7 in, 1 out]
          }
          event "TestCase": Value Change {
            n202 = event-data() -> ()  [unwired: 1 in, 1 out]
            n203 = call "ExEng_TestCases_UpdateGUI.vi"("error in"=w483, "VI ServerCluster"=w481) -> ("error out"=w482:errorcluster)  [unwired: 6 in, 3 out]
          }
          event "TestCase.Add.Instruction": Value Change {
            n204 = event-data() -> ()  [unwired: 1 in, 1 out]
            n205 = call "ExEng_TestCase_Instruction_ADD.vi"("error in"=w486, "VI Server.RefsCluster"=w485) -> ("error out"=w484:errorcluster)  [unwired: 8 in, 1 out]
          }
          event "TestCase.Execute.All": Value Change {
            n206 = event-data() -> ()  [unwired: 1 in, 1 out]
            n207 = call "ExEng_Accessor_Test_ExecuteALL_Ref.vi"() -> ("ExecuteALL"=w487:refnum<queue>)  [unwired: 6 in]
            n208 = Enqueue Element(queue=w487, element=ExcEng_TestCommand."Execute.All", error in (no error)=w489) -> (error out=w490:errorcluster)  [unwired: 1 in, 2 out]
          }
          event "TestCase.Execute.Instruction", "TestCase.Diagnostics.Instruction": Value Change {
            n209 = event-data() -> ()  [unwired: 1 in, 1 out]
            n210 = call "ExEng_Accessor_Test_ExecuteInstruction_Ref.vi"() -> ("ExecuteInstruction"=w491:refnum<queue>)  [unwired: 6 in]
            n211 = Enqueue Element(queue=w491, element=ExcEng_TestCommand."Execute Instruction", error in (no error)=w493) -> (error out=w494:errorcluster)  [unwired: 1 in, 2 out]
          }
          event "TestCase.Execute.Next", "TestCase.Diagnostics.Next": Value Change {
            n212 = event-data() -> ()  [unwired: 1 in, 1 out]
            n213 = call "ExEng_Accessor_TestCase_Execution_Pause_Ref.vi"() -> ("TestCase.Execution.Pause"=w502:refnum<notifier>)  [unwired: 6 in]
            n214 = Send Notification(notification=FALSE, notifier=w502, error in (no error)=w503) -> (notifier out=w496:refnum<notifier>, error out=w500:errorcluster)
            n215 = call "Time Delay"("error in (no error)"=w500, "Delay Time (s)"=0.1) -> ("error out"=w498:errorcluster)  [unwired: 9 in]
            n216 = Send Notification(notification=TRUE, notifier=w496, error in (no error)=w498) -> (error out=w497:errorcluster)  [unwired: 1 out]
          }
          event "TestCase.Execute.Pause", "TestCase.Diagnostics.Pause": Value Change {
            n217 = event-data() -> ("CtlRef"=w506:refnum<vi>, "NewVal"=w504:bool)  [unwired: 1 in]
            n218 = call "ExecEng_GUI_Mngt_PauseTestExecution.vi"("Ctl.Value"=w504, "Ctl.Ref"=w506, "error in (no error)"=w507, "VI Server.RefsCluster"=w505) -> ("error out"=w508:errorcluster)  [unwired: 7 in]
          }
          event "TestCase.Execute.Selected", "TestCase.Execute.All": Shortcut Menu Selection (User) {
            n219 = event-data() -> ("CtlRef"=w511:refnum<vi>)  [unwired: 1 in]
            n220 = property on="Property Node" class="Bool"(reference=w511, error in=w512, "DisabledEnum"=T2."Enabled" ("Disabled")) -> (error out=w510:errorcluster)  [unwired: 1 out]
          }
          event "TestCase.Execute.Selected": Value Change {
            n221 = event-data() -> ()  [unwired: 1 in, 1 out]
            n222 = call "ExEng_Accessor_Test_ExecuteALL_Ref.vi"() -> ("ExecuteALL"=w513:refnum<queue>)  [unwired: 6 in]
            n223 = Enqueue Element(queue=w513, element=ExcEng_TestCommand."Execute.Selected", error in (no error)=w515) -> (error out=w516:errorcluster)  [unwired: 1 in, 2 out]
          }
          event "TestCase.Execute.Step.Pause": Value Change {
            n224 = event-data() -> ()  [unwired: 1 in, 1 out]
            n225 = call "ExEng_Accessor_TestCase_Execution_Pause_Ref.vi"() -> ("TestCase.Execution.Pause"=w520:refnum<notifier>)  [unwired: 6 in]
            n226 = Send Notification(notification=FALSE, notifier=w520, error in (no error)=w519) -> (error out=w518:errorcluster)  [unwired: 1 out]
          }
          event "TestCase.Execution.StepTime": Value Change {
            n227 = event-data() -> ("NewVal"=w521:u32)  [unwired: 1 in]
            n228 = call "ExEng_Accessor_TestCase_Execution_StepTime_Ref.vi"() -> ("TestCase.Execution.StepTime"=w522:refnum<notifier>)  [unwired: 6 in]
            n229 = Send Notification(notification=w521, notifier=w522, error in (no error)=w524) -> (error out=w523:errorcluster)  [unwired: 1 out]
          }
          event "TestCase.Function": Shortcut Menu Activation? {
            n230 = event-data() -> ("MenuRef"=w526:refnum<k9>)  [unwired: 1 in]
            n231 = call "ExEng_Accessor_TestCase_Function.Menu_Ref.vi"() -> ("TestCase.Function.MenuRef"=w527:refnum<notifier>)  [unwired: 6 in]
            n232 = Send Notification(notification=w526, notifier=w527, error in (no error)=w528) -> (error out=w529:errorcluster)  [unwired: 1 out]
            n233 = event-data ("Event Filter Node")("Discard?"=FALSE) -> ()  [unwired: 1 in, 1 out]
          }
          event "TestCase.Function": Shortcut Menu Selection (User) {
            n234 = event-data() -> ("ItemTag"=w530:string)  [unwired: 1 in]
            n235 = call "ExecEng_Function_UserMenu.vi"("ItemTag"=w530, "error in (no error)"=w533, "VI Server.RefsCluster"=w531) -> ("error out"=w532:errorcluster)  [unwired: 8 in]
          }
          event "TestCase.Function": Value Change {
            n236 = event-data() -> ()  [unwired: 1 in, 1 out]
            n237 = call "ExecEng_TestCaseFunction_VaueChanged.vi"("error in (no error)"=w536, "VI Server.RefsCluster"=w535) -> ("error out"=w534:errorcluster)  [unwired: 8 in, 1 out]
          }
          event "TestCase.Function.Argument1": Value Change {
            n238 = event-data() -> ()  [unwired: 1 in, 1 out]
            n239 = call "ExEng_TesdtCaseConfig_Function_Argument2_Populate.vi"("error in"=w539, "VI Server.RefsCluster"=w537) -> ("error out"=w538:errorcluster)  [unwired: 8 in, 1 out]
          }
          event "TestCase.Function.Argument2", "TestCase.Function", "Settings.P/N", "Test.P/N": Mouse Enter {
            n240 = event-data() -> ("CtlRef"=w541:refnum<vi>)  [unwired: 1 in]
            n241 = call "ExecEng_Function_Help.vi"("Control.Ref"=w541, "error in (no error)"=w543, "VI Server Cluster"=w540) -> ("error out"=w542:errorcluster)  [unwired: 8 in]
          }
          event "TestCase.Function.Argument2": Value Change {
            n242 = event-data() -> ()  [unwired: 1 in, 1 out]
            n243 = call "ExEng_TestCaseConfig_Function_Argument3_Populate.vi"("error in"=w546, "VI Server.RefsCluster"=w545) -> ("error out"=w544:errorcluster)  [unwired: 7 in, 2 out]
          }
          event "TestCase.Function.Argument3": Shortcut Menu Selection (User) {
            n244 = event-data() -> ("ItemTag"=w550:string)  [unwired: 1 in]
            n245 = case shown="\"Find All Instances\"" w550 {
              selector: w550 -> [_ _ w568]
              tunnel: w549 -> [w551 w563 w566]
              tunnel: [w551 w557 w565] -> w548
              tunnel: w547 -> [_ w555 w567]
              frame "", Default {
              }
              frame "Get Numbers" {
                n246 = call "ExEng_Accessor_UUT_LimitsFile_Ref.vi"() -> ("UUT.LimitsFile"=w564:refnum<notifier>)  [unwired: 6 in]
                n247 = Get Notifier Status(notifier=w564, error in (no error)=w563) -> (current notification=w561:path, error out=w562:errorcluster)  [unwired: 3 out]
                n248 = call "Configuration_GetSectionNames.vi"("Close File"=TRUE, "error in (no error)"=w562, "Configuration.File.Path"=w561) -> ("error out"=w558:errorcluster, "section names"=w560:string[])  [unwired: 5 in, 2 out]
                n249 = Decimal String To Number(string=w560, default (0L)=u16 0 ("default (0 I32)")) -> (number=w554:u16[])  [unwired: 1 in, 1 out]
                n250 = call-poly "VI Server_SetControl.vi"("Data"=w554, "Control.Label"="Limits.List", "error in"=w558, "SingleInstance"=TRUE, "VI Server.RefsCluster"=w555) -> ("error out"=w557:errorcluster)  [unwired: 4 in, 2 out]
              }
              frame "Find All Instances" {
                n251 = call "ExecEng_Memory_CheckForConflicts.vi"("ItemTag"=w568, "error in (no error)"=w566, "VI Server.RefsCluster"=w567) -> ("error out"=w565:errorcluster)  [unwired: 8 in]
              }
            }
          }
          event "TestCase.Function.Argument3": Value Change {
            n252 = event-data() -> ()  [unwired: 1 in, 1 out]
            n253 = call "ExecEng_NumMem_CheckForConcistency.vi"("error in (no error)"=w571, "VI Server.RefsCluster"=w570) -> ("error out"=w569:errorcluster)  [unwired: 9 in]
          }
          event "TestCase.Instrument.Data": Shortcut Menu Selection (User) {
            n254 = event-data() -> ("ItemTag"=w574:string)  [unwired: 1 in]
            n255 = case shown="\"Clear Data\"" w574 {
              tunnel: w575 -> [w576 w582]
              tunnel: w573 -> [_ w581]
              tunnel: [w576 w579] -> w572
              frame "False", Default {
              }
              frame "Clear Data" {
                n256 = call-poly "VI Server_SetControl.vi"("Data"=0.0, "Control.Label"="TestCase.Instrument.Data", "error in"=w582, "SingleInstance"=TRUE, "VI Server.RefsCluster"=w581) -> ("error out"=w579:errorcluster)  [unwired: 4 in, 2 out]
              }
            }
          }
          event "TestCase.LimitsIndex": Shortcut Menu Selection (User) {
            n257 = event-data() -> ("ItemTag"=w583:string)  [unwired: 1 in]
            n258 = call "ExecEng_Limit_CheckForConflicts.vi"("ItemTag"=w583, "error in (no error)"=w586, "VI Server.RefsCluster"=w585) -> ("error out"=w584:errorcluster)  [unwired: 8 in]
          }
          event "TestCase.LimitsIndex": Value Change {
            n259 = event-data() -> ()  [unwired: 1 in, 1 out]
            n260 = call "ExEng_TesdtCaseConfig_Limits_ValueChanged.vi"("error in"=w589, "VI Server.RefsCluster"=w588) -> ("error out"=w587:errorcluster)  [unwired: 8 in, 1 out]
          }
          event "TestCase.SAVE": Value Change {
            n261 = event-data() -> ()  [unwired: 1 in, 1 out]
            n262 = call "ExEng_TestCase_SAVE.vi"("error in"=w592, "VI Server.RefsCluster"=w590) -> ("error out"=w591:errorcluster)  [unwired: 8 in, 1 out]
          }
          event "TestCase.TraceLimits": Value Change {
            n263 = event-data() -> ("NewVal"=w594:bool)  [unwired: 1 in]
            n264 = call "ExEng_Accessor_TestCase_TraceLimits_Ref.vi"() -> ("TestCase.TraceLimits"=w593:refnum<notifier>)  [unwired: 6 in]
            n265 = Send Notification(notification=w594, notifier=w593, error in (no error)=w596) -> (error out=w595:errorcluster)  [unwired: 1 out]
          }
          event "TestCase.Update.Instruction": Value Change {
            n266 = event-data() -> ()  [unwired: 1 in, 1 out]
            n267 = call "ExEng_TestCase_Instruction_UPDATE.vi"("error in"=w599, "VI Server.RefsCluster"=w597) -> ("error out"=w598:errorcluster)  [unwired: 8 in, 1 out]
          }
          event "TestCaseConfiguration": Double Click {
            n268 = event-data() -> ()  [unwired: 1 in, 1 out]
            n269 = call "ExEng_TestCase_Instruction_ExtractFromTestCase.vi"("error in"=w602, "VI Server.RefsCluster"=w600) -> ("error out"=w601:errorcluster)  [unwired: 8 in, 1 out]
          }
          event "TestCaseConfiguration": Shortcut Menu Selection (User) {
            n270 = event-data() -> ("ItemTag"=w603:string)  [unwired: 1 in]
            n271 = call "ExcEng_TestCaseConfig_UserMenu.vi"("ItemTag"=w603, "error in (no error)"=w606, "VI Server.RefsCluster"=w604) -> ("error out"=w605:errorcluster)  [unwired: 8 in]
          }
          event "TestCaseConfiguration": Value Change {
            n272 = event-data() -> ()  [unwired: 1 in, 1 out]
            n273 = call "ExEng_TestCase_Configuration_ValueChanged.vi"("error in"=w609, "VI Server.RefsCluster"=w608) -> ("error out"=w607:errorcluster)  [unwired: 8 in, 1 out]
          }
          event "TestCaseConfiguration_VisibleRow_Decr": Value Change {
            n274 = event-data() -> ()  [unwired: 1 in, 1 out]
            n275 = property on="TestCaseConfiguration" class="MCListbox (strict)"(error in=w615) -> (error out=w614:errorcluster, "TopLeft"=w613:T8)  [unwired: 1 in, 1 out]
            n276 = Unbundle By Name(w613) -> ("Row"=w612:u32)
            n277 = Decrement(x=w612) -> (x-1=w610:u32)
            n278 = case shown="4294967295" w610 {
              selector: w610 -> [w616 _]
              tunnel: w614 -> [w620 w621]
              tunnel: w613 -> [w619 _]
              tunnel: [w617 w621] -> w611
              frame 0, Default {
                n279 = Bundle By Name(cluster=w619, "Row"=w616) -> (w618:T8)
                n280 = property on="TestCaseConfiguration" class="MCListbox (strict)"(error in=w620, "TopLeft"=w618) -> (error out=w617:errorcluster)  [unwired: 1 in, 1 out]
              }
              frame -1 {
              }
            }
          }
          event "TestCaseConfiguration_VisibleRow_Incr": Value Change {
            n281 = event-data() -> ()  [unwired: 1 in, 1 out]
            n282 = property on="TestCaseConfiguration" class="MCListbox (strict)"(error in=w628) -> (error out=w627:errorcluster, "TopLeft"=w626:T8)  [unwired: 1 in, 1 out]
            n283 = Unbundle By Name(w626) -> ("Row"=w625:u32)
            n284 = Increment(x=w625) -> (x+1=w624:u32)
            n285 = Bundle By Name(cluster=w626, "Row"=w624) -> (w623:T8)
            n286 = property on="TestCaseConfiguration" class="MCListbox (strict)"(error in=w627, "TopLeft"=w623) -> (error out=w622:errorcluster)  [unwired: 1 in, 1 out]
          }
          event "TestCaseExecution.PauseOnFailure": Value Change {
            n287 = event-data() -> ("NewVal"=w630:bool)  [unwired: 1 in]
            n288 = call "ExEng_Accessor_TestExecution_Pause_Ref.vi"() -> ("Test.Execution.Pause"=w629:refnum<notifier>)  [unwired: 6 in]
            n289 = Send Notification(notification=w630, notifier=w629, error in (no error)=w631) -> (error out=w632:errorcluster)  [unwired: 1 out]
          }
          event "TestConfiguration": Double Click {
            n290 = event-data() -> ("Row"=w633:i32)  [unwired: 1 in]
            n291 = call "ExcEng_TestConfig_DoubleClick.vi"("Row"=w633, "error in (no error)"=w636, "VI Server.RefsCluster"=w634) -> ("error out"=w635:errorcluster)  [unwired: 8 in]
          }
          event "TestConfiguration": Shortcut Menu Selection (User) {
            n292 = event-data() -> ("ItemTag"=w647:string, "CtlRef"=w646:refnum<vi>)  [unwired: 1 in]
            n293 = call "VI Server_Defer FP Update.vi"("Defer Panel Updates? (F)"=TRUE, "error in"=w644, "VI Server Cluster"=w643) -> ("error out"=w645:errorcluster, "VI Server Cluster.DUP"=w638:T3)  [unwired: 7 in]
            n294 = call "ExecEng_TestConfiguration_UserMenu.vi"("CtlRef"=w646, "ItemTag"=w647, "error in (no error)"=w645, "VI Server.RefsCluster"=w638) -> ("error out"=w641:errorcluster, "VI Server.RefsCluster.DUP"=w637:T3)  [unwired: 6 in]
            n295 = call "VI Server_Defer FP Update.vi"("Defer Panel Updates? (F)"=FALSE, "error in"=w641, "VI Server Cluster"=w637) -> ("error out"=w640:errorcluster)  [unwired: 7 in, 1 out]
          }
          event "TestConfiguration": Value Change {
            n296 = event-data() -> ()  [unwired: 1 in, 1 out]
            n297 = call "ExecEng_TestConfiguration_ValueChanged.vi"("error in (no error)"=w648, "VI Server.RefsCluster"=w650) -> ("error out"=w649:errorcluster)  [unwired: 8 in, 1 out]
          }
          event "TestConfiguration.Run.Step": Value Change {
            n298 = event-data() -> ()  [unwired: 1 in, 1 out]
            n299 = call "ExecEng_Test_LaunchStep.vi"("error in (no error)"=w653, "VI Server.RefsCluster"=w651) -> ("error out"=w652:errorcluster)  [unwired: 9 in]
          }
          event "TestConfiguration.RunAll": Value Change {
            n300 = event-data() -> ()  [unwired: 1 in, 1 out]
            n301 = call "ExEng_Accessor_Test_Command_Ref.vi"() -> ("Test.Command"=w659:refnum<queue>)  [unwired: 6 in]
            n302 = call "ExEng_Accessor_TestCase_Execution_ABORT_Ref.vi"() -> ("TestCase.Execution.ABORT"=w657:refnum<notifier>)  [unwired: 6 in]
            n303 = Enqueue Element(queue=w659, element=ExcEng_TestCommand."TestConfiguration.RunAll", error in (no error)=w660) -> (error out=w656:errorcluster)  [unwired: 1 in, 2 out]
            n304 = Send Notification(notification=FALSE, notifier=w657, error in (no error)=w656) -> (error out=w655:errorcluster)  [unwired: 1 out]
          }
          event "TestExecution.DoNotCheckInstrument": Value Change {
            n305 = event-data() -> ("NewVal"=w663:bool)  [unwired: 1 in]
            n306 = call "ExEng_Accessor_DoNotCheckInstrument_Ref.vi"() -> ("DoNotCheckInstrument"=w662:refnum<notifier>)  [unwired: 6 in]
            n307 = Send Notification(notification=w663, notifier=w662, error in (no error)=w664) -> (error out=w661:errorcluster)  [unwired: 1 out]
          }
          event "TestExecution.PauseInInstrumentsFailure": Value Change {
            n308 = event-data() -> ("NewVal"=w665:bool)  [unwired: 1 in]
            n309 = call "ExEng_Accessor_TestExecution.PauseInInstrumentsFailure_Ref.vi"() -> ("TestExecution.PauseInInstrumentsFailure"=w667:refnum<notifier>)  [unwired: 6 in]
            n310 = Send Notification(notification=w665, notifier=w667, error in (no error)=w668) -> (error out=w666:errorcluster)  [unwired: 1 out]
          }
          event "TestTree.CollapseItems": Value Change {
            n311 = event-data() -> ("NewVal"=w670:bool)  [unwired: 1 in]
            n312 = call "ExEng_Accessor_TestTree_Collapse_Items_Ref.vi"() -> ("TestTree.CollapseItems"=w669:refnum<notifier>)  [unwired: 6 in]
            n313 = Send Notification(notification=w670, notifier=w669, error in (no error)=w672) -> (error out=w671:errorcluster)  [unwired: 1 out]
          }
          event "UDP.IP.Address": Value Change {
            n314 = event-data() -> ("NewVal"=w675:string, "OldVal"=w674:string)  [unwired: 1 in]
            n315 = call "ExEng_UDP_CheckMulticast_IP_Address.vi"("Old.IP.Address"=w674, "New.IP.Address"=w675, "error in"=w676, "VI Server.RefsCluster"=w677) -> ("error out"=w673:errorcluster)  [unwired: 6 in, 1 out]
          }
          event "UDP.LocalPort": Value Change {
            n316 = event-data() -> ("NewVal"=w679:u16)  [unwired: 1 in]
            n317 = call "ExEng_Accessor_UDP_LocalPort_Ref.vi"() -> ("UDP.LocalPort"=w680:refnum<notifier>)  [unwired: 6 in]
            n318 = Send Notification(notification=w679, notifier=w680, error in (no error)=w681) -> (error out=w678:errorcluster)  [unwired: 1 out]
          }
          event "UDP.Port.BC": Value Change {
            n319 = event-data() -> ("NewVal"=w684:u16)  [unwired: 1 in]
            n320 = call "ExEng_Accessor_UDP_Port_Read_Ref.vi"() -> ("UDP.Port.BC"=w682:refnum<notifier>)  [unwired: 6 in]
            n321 = Send Notification(notification=w684, notifier=w682, error in (no error)=w685) -> (error out=w683:errorcluster)  [unwired: 1 out]
          }
          event "UDP.Port.RT": Value Change {
            n322 = event-data() -> ("NewVal"=w688:u16)  [unwired: 1 in]
            n323 = call "ExEng_Accessor_UDP_Port_Receiver_Ref.vi"() -> ("UDP.Port.RT"=w686:refnum<notifier>)  [unwired: 6 in]
            n324 = Send Notification(notification=w688, notifier=w686, error in (no error)=w689) -> (error out=w687:errorcluster)  [unwired: 1 out]
          }
          event "UDP.Responce.Array": Shortcut Menu Selection (User) {
            n325 = event-data() -> ("ItemTag"=w690:string)  [unwired: 1 in]
            n326 = case shown="\"Clear\"" w690 {
              tunnel: w693 -> [w694 w700]
              tunnel: [w694 w699] -> w692
              tunnel: w691 -> [_ w698]
              frame "False", Default {
              }
              frame "Clear" {
                n327 = call-poly "VI Server_SetControl.vi"("Data"=string[] [], "Control.Label"="UDP.Responce.Array", "error in"=w700, "SingleInstance"=TRUE, "VI Server.RefsCluster"=w698) -> ("error out"=w699:errorcluster)  [unwired: 4 in, 2 out]
              }
            }
          }
          event "UDP.Responce.Array.EmptyAtStart": Value Change {
            n328 = event-data() -> ("NewVal"=w702:bool)  [unwired: 1 in]
            n329 = call "ExEng_Accessor_UDP_Responce_Array_EmptyAtStart_Ref.vi"() -> ("UDP.Responce.Array.EmptyAtStart"=w703:refnum<notifier>)  [unwired: 6 in]
            n330 = Send Notification(notification=w702, notifier=w703, error in (no error)=w704) -> (error out=w701:errorcluster)  [unwired: 1 out]
          }
          event "UDP.Responce.String.Monitor": Value Change {
            n331 = event-data() -> ("NewVal"=w706:bool)  [unwired: 1 in]
            n332 = call "ExEng_Accessor_UDP_Responce_String_Monitor_Ref.vi"() -> ("UDP.Responce.String.Monitor"=w709:refnum<notifier>)  [unwired: 6 in]
            n333 = Send Notification(notification=w706, notifier=w709, error in (no error)=w710) -> (error out=w708:errorcluster)  [unwired: 1 out]
            n334 = case shown="False" w706 {
              tunnel: w708 -> [w716 w717]
              tunnel: [w715 w717] -> w705
              tunnel: w707 -> [w714 _]
              frame False {
                n335 = call-poly "VI Server_SetControl.vi"("Data"=string[] [], "Control.Label"="UDP.Responce.Array", "error in"=w716, "SingleInstance"=TRUE, "VI Server.RefsCluster"=w714) -> ("error out"=w715:errorcluster)  [unwired: 4 in, 2 out]
              }
              frame True {
              }
            }
          }
          event "UDP.Test.String.Send": Value Change {
            n336 = event-data() -> ()  [unwired: 1 in, 1 out]
            n337 = call-poly "VI Server_GetControl_Value_Ref.vi"("DataType"="" ("Empty String Constant"), "Control.Label"="UDP.Test.String", "error in"=w724, "SingleInstance"=TRUE, "VI Server.RefsCluster"=w723) -> ("error out"=w725:errorcluster, "Value"=w719:string)  [unwired: 3 in, 2 out]
            n338 = call "ExEng_Accessor_UDP_Instrument_Instruction_Ref.vi"() -> ("UDP.Instrument.Instruction"=w726:refnum<queue>)  [unwired: 6 in]
            n339 = Enqueue Element(queue=w726, element=w719, error in (no error)=w725) -> (error out=w718:errorcluster)  [unwired: 1 in, 2 out]
          }
          event "UDP.Test.String2.Send": Value Change {
            n340 = event-data() -> ()  [unwired: 1 in, 1 out]
            n341 = call-poly "VI Server_GetControl_Value_Ref.vi"("DataType"="" ("Empty String Constant"), "Control.Label"="UDP.Test.String2", "error in"=w733, "SingleInstance"=TRUE, "VI Server.RefsCluster"=w732) -> ("error out"=w734:errorcluster, "Value"=w728:string)  [unwired: 3 in, 2 out]
            n342 = call "ExEng_Accessor_UDP_Instrument_Instruction_Ref.vi"() -> ("UDP.Instrument.Instruction"=w735:refnum<queue>)  [unwired: 6 in]
            n343 = Enqueue Element(queue=w735, element=w728, error in (no error)=w734) -> (error out=w727:errorcluster)  [unwired: 1 in, 2 out]
          }
          event "UDP.Write.Array": Shortcut Menu Selection (User) {
            n344 = event-data() -> ("ItemTag"=w736:string)  [unwired: 1 in]
            n345 = case shown="\"Clear\"" w736 {
              tunnel: w739 -> [w740 w749]
              tunnel: [w740 w743] -> w738
              tunnel: w737 -> [_ w748]
              frame "False", Default {
              }
              frame "Clear" {
                n346 = call-poly "VI Server_SetControl.vi"("Data"=string[] [], "Control.Label"="UDP.Write.Array", "error in"=w749, "SingleInstance"=TRUE, "VI Server.RefsCluster"=w748) -> ("error out"=w744:errorcluster, "Control.Ref"=w742:refnum<vi>)  [unwired: 4 in, 1 out]
                n347 = property on="Property Node" class="Arr (strict)"(reference=w742, error in=w744, "Index Values"=u32[] [0]) -> (error out=w743:errorcluster)  [unwired: 1 out]
              }
            }
          }
          event "User.AddNew": Value Change {
            n348 = event-data() -> ()  [unwired: 1 in, 1 out]
            n349 = call "ExecEng_Login_Users_Add.vi"("error in (no error)"=w752, "VI Server.RefsCluster"=w750) -> ("error out"=w751:errorcluster)  [unwired: 9 in]
          }
          event "User.Remove": Value Change {
            n350 = event-data() -> ()  [unwired: 1 in, 1 out]
            n351 = call "ExecEng_Login_Users_Remove.vi"("error in (no error)"=w755, "VI Server.RefsCluster"=w754) -> ("error out"=w753:errorcluster)  [unwired: 9 in]
          }
          event "User.SAVE": Value Change {
            n352 = event-data() -> ()  [unwired: 1 in, 1 out]
            n353 = call "ExecEng_Login_Users_Save.vi"("error in (no error)"=w758, "VI Server.RefsCluster"=w756) -> ("error out"=w757:errorcluster)  [unwired: 9 in]
          }
          event "Users": Value Change {
            n354 = event-data() -> ()  [unwired: 1 in, 1 out]
            n355 = call "ExecEng_Login_Users_ValueChanged.vi"("error in (no error)"=w761, "VI Server.RefsCluster"=w760) -> ("error out"=w759:errorcluster)  [unwired: 9 in]
          }
          event "Users.Load": Value Change {
            n356 = event-data() -> ()  [unwired: 1 in, 1 out]
            n357 = call "ExecEng_Login_Users_Load.vi"("error in (no error)"=w764, "VI Server.RefsCluster"=w762) -> ("error out"=w763:errorcluster)  [unwired: 9 in]
          }
          event Menu Activation? {
            n358 = event-data() -> ()  [unwired: 1 in, 1 out]
            n359 = event-data ("Event Filter Node")() -> ()  [unwired: 2 in, 1 out]
          }
          event Menu Selection (User) {
            n360 = event-data() -> ("ItemTag"=w766:string)  [unwired: 1 in]
            n361 = call "ExEng_MainVI_UserMenu_Selection.vi"("Menu.ItemTag"=w766, "error in"=w768, "VI Server.RefsCluster"=w767) -> ("error out"=w769:errorcluster)  [unwired: 7 in, 1 out]
          }
          event Timeout {
            n362 = event-data() -> ()  [unwired: 1 in, 1 out]
            n363 = call "ExEng_UserLastSelection_Set_Get.vi"("LoopCounter"=w772, "SynchRefs.Set/Get"=SynchRefs_SetGet."Set", "error in"=w775, "VI Server.RefsCluster"=w774) -> ("error out"=w770:errorcluster)  [unwired: 6 in, 1 out]
            n364 = First Call?() -> (First Call?: T/F=w771:bool)
            n365 = case shown="True" w771 {
              frame False {
              }
              frame True {
                n366 = Control Help Window(1:FALSE ("Show")) -> ()  [unwired: 1 in]
              }
            }
          }
          event "CurrentInstruction": Shortcut Menu Selection (User) {
            n367 = event-data() -> ("ItemTag"=w780:string)  [unwired: 1 in]
            n368 = case shown="\"Open Instrument Soft Panel\"" w780 {
              tunnel: w779 -> [w781 w784]
              tunnel: [w781 w782] -> w778
              tunnel: w777 -> [_ w783]
              frame "False", Default {
              }
              frame "Open Instrument Soft Panel" {
                n369 = call "ExecEng_CurrentInstruction_Instrument_Open.vi"("error in (no error)"=w784, "VI Server.RefsCluster"=w783) -> ("error out"=w782:errorcluster)  [unwired: 9 in]
              }
            }
          }
        }
        n370 = call "ExEng_Accessor_EXIT_Ref.vi"() -> ("EXIT"=w54:refnum<notifier>)  [unwired: 6 in]
        n371 = call "StopOnErrorOrCommand.vi"("STOP"=w54, "error in (no error)"=w56) -> ("error out"=w57:errorcluster, "STOP"=w55:bool)  [unwired: 8 in]
      }
      n372 = call "ExecEng_UDP_MAIN.vi"("error in (no error)"=w19, "VI Server.RefsCluster"=w20) -> ("error out"=w24:errorcluster)  [unwired: 9 in]
      n373 = while {
        tunnel: w19 -> [w35]
        tunnel: [w30] -> w21
        tunnel: w20 -> [w29]
        stop <- w28 stop-if-true
        n374 = flat-sequence {
          tunnel: w35 -> [w50]
          tunnel: [w50] -> w33
          frame #0 {
          }
        }
        n375 = event shown="[0] Timeout" {
          selector: _ -> [_ _]
          dyn-events: _ -> [_ _]
          timeout: 250 -> [_ _]
          tunnel: w33 -> [w38 w47]
          tunnel: [w36 w44] -> w31
          tunnel: w29 -> [w37 w43]
          event Timeout {
            n376 = event-data() -> ()  [unwired: 1 in, 1 out]
            n377 = disable-structure "Diagram Disable Structure" shown="Disabled" {
              disable-tunnel: [w41 w42] -> w36
              disable-tunnel: w38 -> [w40 w42]
              disable-tunnel: w37 -> [w39 _]
              frame Disabled {
                n378 = call "ExecEng_CodeTest.vi"("error in"=w40, "VI Server.RefsCluster"=w39) -> ("error out"=w41:errorcluster)  [unwired: 9 in]
              }
              frame Enabled {
              }
            }
          }
          event "EXIT": Value Change {
            n379 = event-data() -> ()  [unwired: 1 in, 1 out]
            n380 = call "ExecEng_Instruments_EXIT.vi"("error in (no error)"=w47, "VI Server.RefsCluster"=w43) -> ("error out"=w46:errorcluster)  [unwired: 8 in, 1 out]
            n381 = call "ExEng_Accessor_EXIT_Ref.vi"() -> ("EXIT"=w48:refnum<notifier>)  [unwired: 6 in]
            n382 = Send Notification(notification=TRUE, notifier=w48, error in (no error)=w46) -> (error out=w45:errorcluster)  [unwired: 1 out]
            n383 = call "ExEng_EXIT_Main.vi"("error in"=w45, "VI Server.RefsCluster"=w43) -> ("error out"=w44:errorcluster)  [unwired: 8 in, 1 out]
          }
        }
        n384 = call "ExEng_Accessor_EXIT_Ref.vi"() -> ("EXIT"=w32:refnum<notifier>)  [unwired: 6 in]
        n385 = call "StopOnErrorOrCommand.vi"("STOP"=w32, "error in (no error)"=w31) -> ("error out"=w30:errorcluster, "STOP"=w28:bool)  [unwired: 8 in]
      }
      n386 = call "ExecEng_TEST_MAIN.vi"("error in (no error)"=w19, "VI Server.RefsCluster"=w20) -> ("error out"=w22:errorcluster)  [unwired: 9 in]
      n387 = call "ExecEng_TEST_ExecuteALL.vi"("error in (no error)"=w19, "VI Server.RefsCluster"=w20) -> ("error out"=w18:errorcluster)  [unwired: 9 in]
      n388 = call "ExecEng_TEST_ExecuteInstruction.vi"("error in (no error)"=w19, "VI Server.RefsCluster"=w20) -> ("error out"=w17:errorcluster)  [unwired: 9 in]
      n389 = Build Array(w21, w17, w18, w22, w24) -> (w23:errorcluster[])
      n390 = call "Merge Errors II.vi"("error array in"=w23, "error in 1 (no error)"=w26) -> ("error out.DUP"=w25:errorcluster)  [unwired: 4 in, 1 out]
    }
    frame Error {
    }
  }
  n391 = call "VI Server_CloseRefs.vi"("error in"=w1, "VI Server.RefsCluster"=w9) -> ("error out"=w12:errorcluster)  [unwired: 9 in]
  n392 = call "ExEng_Synch_CLOSE.vi"("error in"=w12) -> ("error out"=w4:errorcluster)  [unwired: 10 in]
  n393 = Current VI's Path() -> (path=w5:path)
  n394 = call "Close Window If in EXE mode.vi"("TopLevelVI Path"=w5, "error in"=w4) -> ("error out"=→"error out":errorcluster)  [unwired: 9 in]
  n395 = call <vilib>:"Simple Error Handler.vi"("error in (no error)"=w4) -> ()  [unwired: 4 in, 5 out]
